vi "SISE-Monitor110.vi"() -> ()   [LabVIEW 2024]
uses:
  Labview-Projects2019/IonFluxProgramms2019/IonFluxMonitor/SubVIs-SISE-Monitor/Control-IonFlux.ctl
  <vilib>/DAQmx/read.llb/DAQmx Read (Analog 2D DBL NChan NSamp).vi
  <vilib>/Instr/_visa.llb/VISA Configure Serial Port (Instr).vi
  <vilib>/DAQmx/create/channels.llb/DAQmx Create Channel (AI-Voltage-Basic).vi
  <vilib>/DAQmx/miscellaneous.llb/DAQmx Fill In Error Info.vi
  <vilib>/Analysis/NI_AALPro.lvlib
panel:
  out "Lesepuffer":string
  out "Registerkarte":enum32{"Start", "Record", "Stop"}(tab)
  out "Output V ch 2":bool
  in  "V channel 2":bool
  out "Output V ch 1":bool
  in  "V channel 1":bool
  out "SISE channel 1":bool
  out "Output SISE ch 2":bool
  in  "SISE channel 2":bool
  out "slow":bool
  in  "Scan angle (degrees)":dbl(slide) scale=0.0..90.0
  out "?":dbl
  in  "VISA res. name":refnum<visa-resource-name> caption="VISA-Ressourcenname"
  in  "Start measurement":bool
  out "Data File":bool
  out "Ind. Channel In":bool
  in  "Data file":path
  out "Ind. Channel Out":bool
  out "?":dbl
  out "Record period (round at 5s)":dbl
  in  "Scan distance (µm)":dbl(slide)=50.0 scale=0.0..100.0
  in  "Record period (single track, s)":dbl(slide)=10.112359550561797 scale=0.0..60.0 scale format="%#_2f"
  in  "Manipulator Speed":bool
  out "fast":bool
  in  "Channels In":tag
  in  "Position of manipulator":bool=TRUE
  out "right":bool
  out "left":bool
  in  "TC 3":T1(tab)
  in  "Range limit\nS1.1 (mV)":dbl(slide)=200.0 min=0.0 max=600.0 scale=0.2..600.0
  in  "Base line\nS1.1 (mV)":dbl(slide) scale=-300.0..300.0
  in  "Range limit\nS1.2 mV":dbl(slide)=30.0 scale=0.1..30.0
  in  "Base line \nS1.2 (mV)":dbl(slide) scale=-15.0..15.0
  out "dV-SISE channel 1":cluster{dbl[], dbl[]}[](graph)
  out "V-SISE channel 1":cluster{dbl[], dbl[]}[](graph)
  out "V-SISE channel 2":cluster{dbl[], dbl[]}[](graph)
  out "dV-SISE channel 2":cluster{dbl[], dbl[]}[](graph)
  in  "Range limit\nS2.1 (mV)":dbl(slide)=200.0 min=0.0 max=600.0 scale=0.2..600.0
  in  "Base line\nS2.1 (mV)":dbl(slide) scale=-300.0..300.0
  in  "Base line \nS2.2 (mV)":dbl(slide) scale=-15.0..15.0
  in  "Range limit\nS2.2 (mV)":dbl(slide)=30.0 scale=0.1..30.0
  out "Voltage channel 1":cluster{dbl[], dbl[]}[](graph)
  in  "Base line\nV1 (V)":dbl(slide) scale=-10.0..10.0
  in  "Range limit\nV1 (V)":dbl(slide)=24.63054187192118 min=0.0 max=600.0 scale=0.0..25.0
  in  "Base line\nV2 (V)":dbl(slide) scale=-10.0..10.0
  in  "Range limit\nV2 (V)":dbl(slide)=24.63054187192118 min=0.0 max=600.0 scale=0.0..25.0
  out "Voltage channel 2":cluster{dbl[], dbl[]}[](graph)
  out "V channel #2":bool
  out "V channel #1":bool
  out "SISE channel #2":bool
  out "SISE channel #1":bool
  in  "?":T2(tab)
  out "Vprobe SISE 1":cluster{dbl[], dbl[]}[](graph)
  out "Vprobe SISE 2":cluster{dbl[], dbl[]}[](graph)
  out "Vprobe V 1":cluster{dbl[], dbl[]}[](graph)
  out "Vprobe V 2":cluster{dbl[], dbl[]}[](graph)
  in  "Enable change position 0":bool
  out "Raw data file":path
  in  "Stop measurent":bool
  out "Position probe":cluster{dbl[], dbl[]}[](graph)
  in  "Add Mark":bool
  in  "Event Mark":string
  out "Stop recording":bool
  out "String":string
  out "E-mark on":T3
  out "?":string
  in  "Bildlaufleiste":i32(c297)
  in  "Start fit (% of rec. period)":dbl(slide)=50.0 scale=0.0..100.0
  in  "?":enum32{"dV SISE 1", "dV SISE 2"}(tab)
  out "deltaV SISE 1":cluster{dbl[], "Best Linear Fit":dbl[]}[](graph)
  out "deltaV SISE 2":cluster{dbl[], "Best Linear Fit":dbl[]}[](graph)
  in  "Zoom from start":dbl(slide) scale=0.0..100.0
  in  "Zoom from end":dbl(slide)=100.0 scale=0.0..100.0
  in  "Stop programm":bool
  in  "New measurement":bool
  out "Stop recording 2":bool
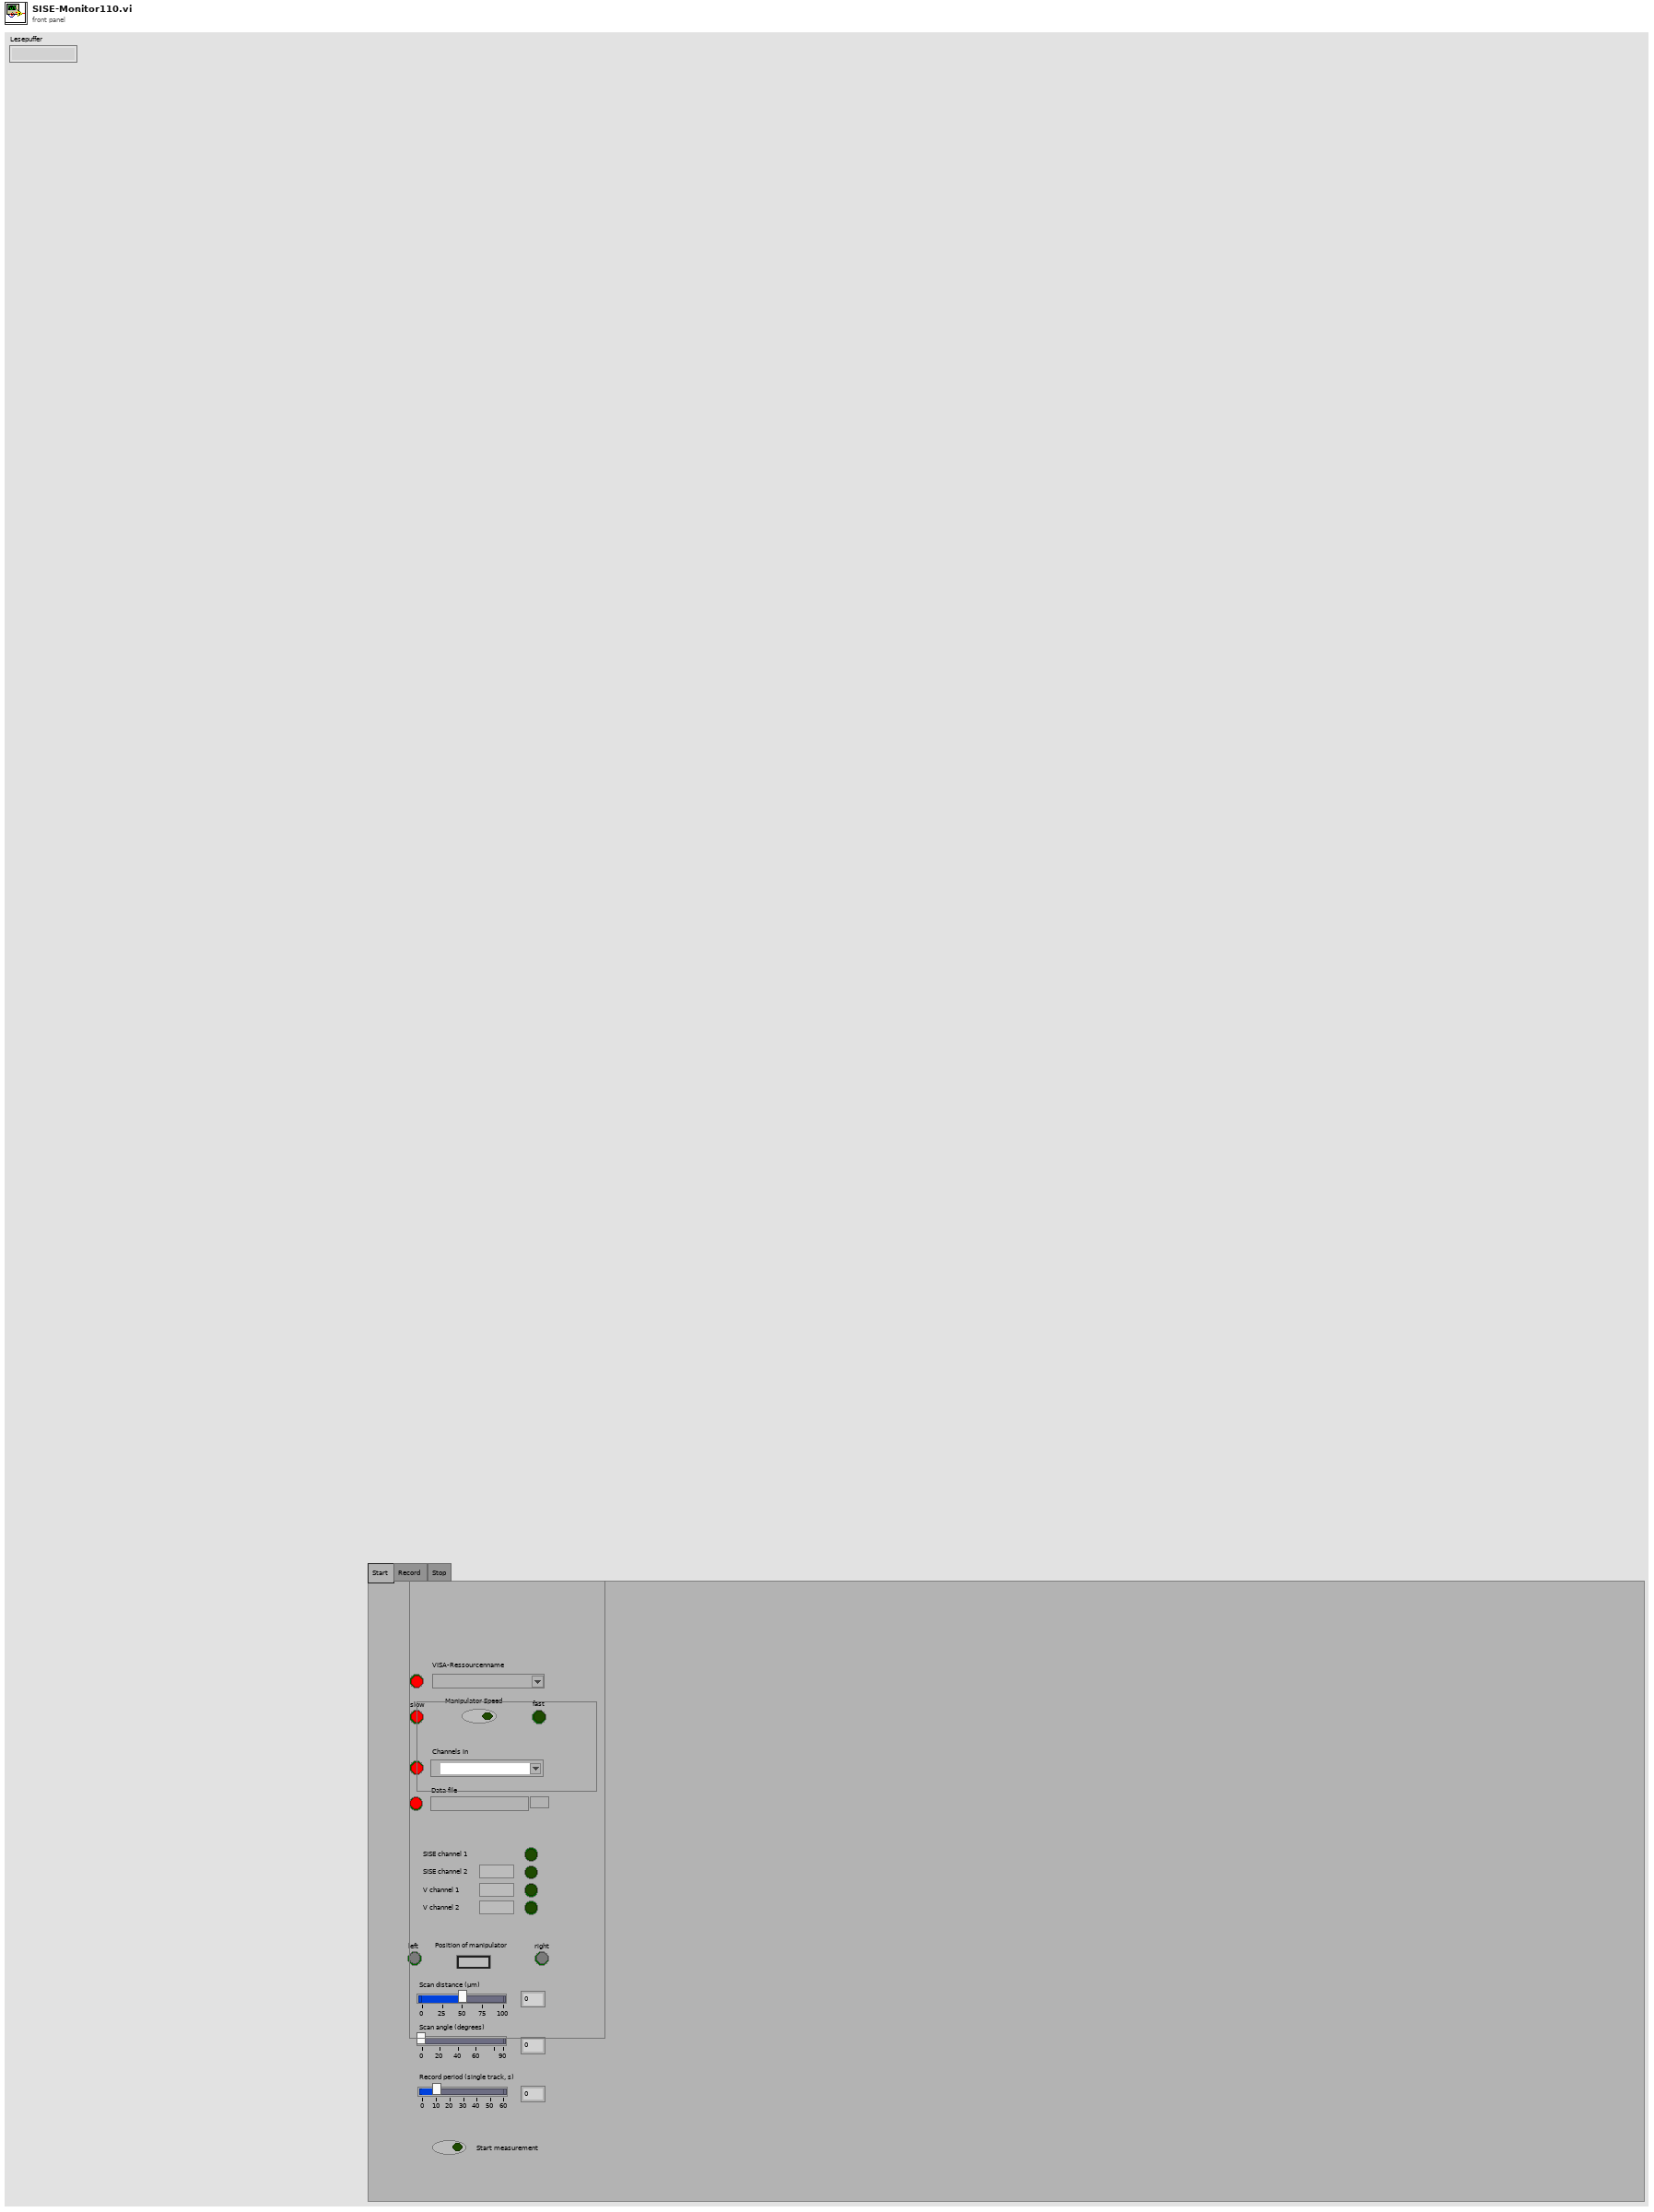
[diagram p1: front panel]
types:
  T1 = enum32{"SISE channel #1", "SISE channel #2", "V channel #1", "V channel #2"}
  T2 = enum32{"SISE chan #1", "SISE chan #2", "V chan #1", "V chan #2"}
  T3 = typedef "Control-IonFlux.ctl" = bool
  T4 = cluster{"refnum out":refnum<file>, "status":bool, "code":i32, "source":string}
  T5 = cluster{"task out":refnum<k21>, "status":bool, "code":i32, "source":string}
  T6 = enum16{"open", "replace", "create", "open or create", "replace or create", "replace or create with confirmation"}
  T7 = cluster{"refnum":refnum<file>, "status":bool, "code":i32, "source":string}
  T8 = cluster{dbl[], dbl[], "Best Linear Fit":dbl[], dbl[], dbl[]}
  T9 = cluster{"Array (Ausgang)":dbl[], "Array (Ausgang)":dbl[]}
  T10 = cluster{"Array (Ausgang)":dbl[], "Array (Ausgang)":dbl[]}[]
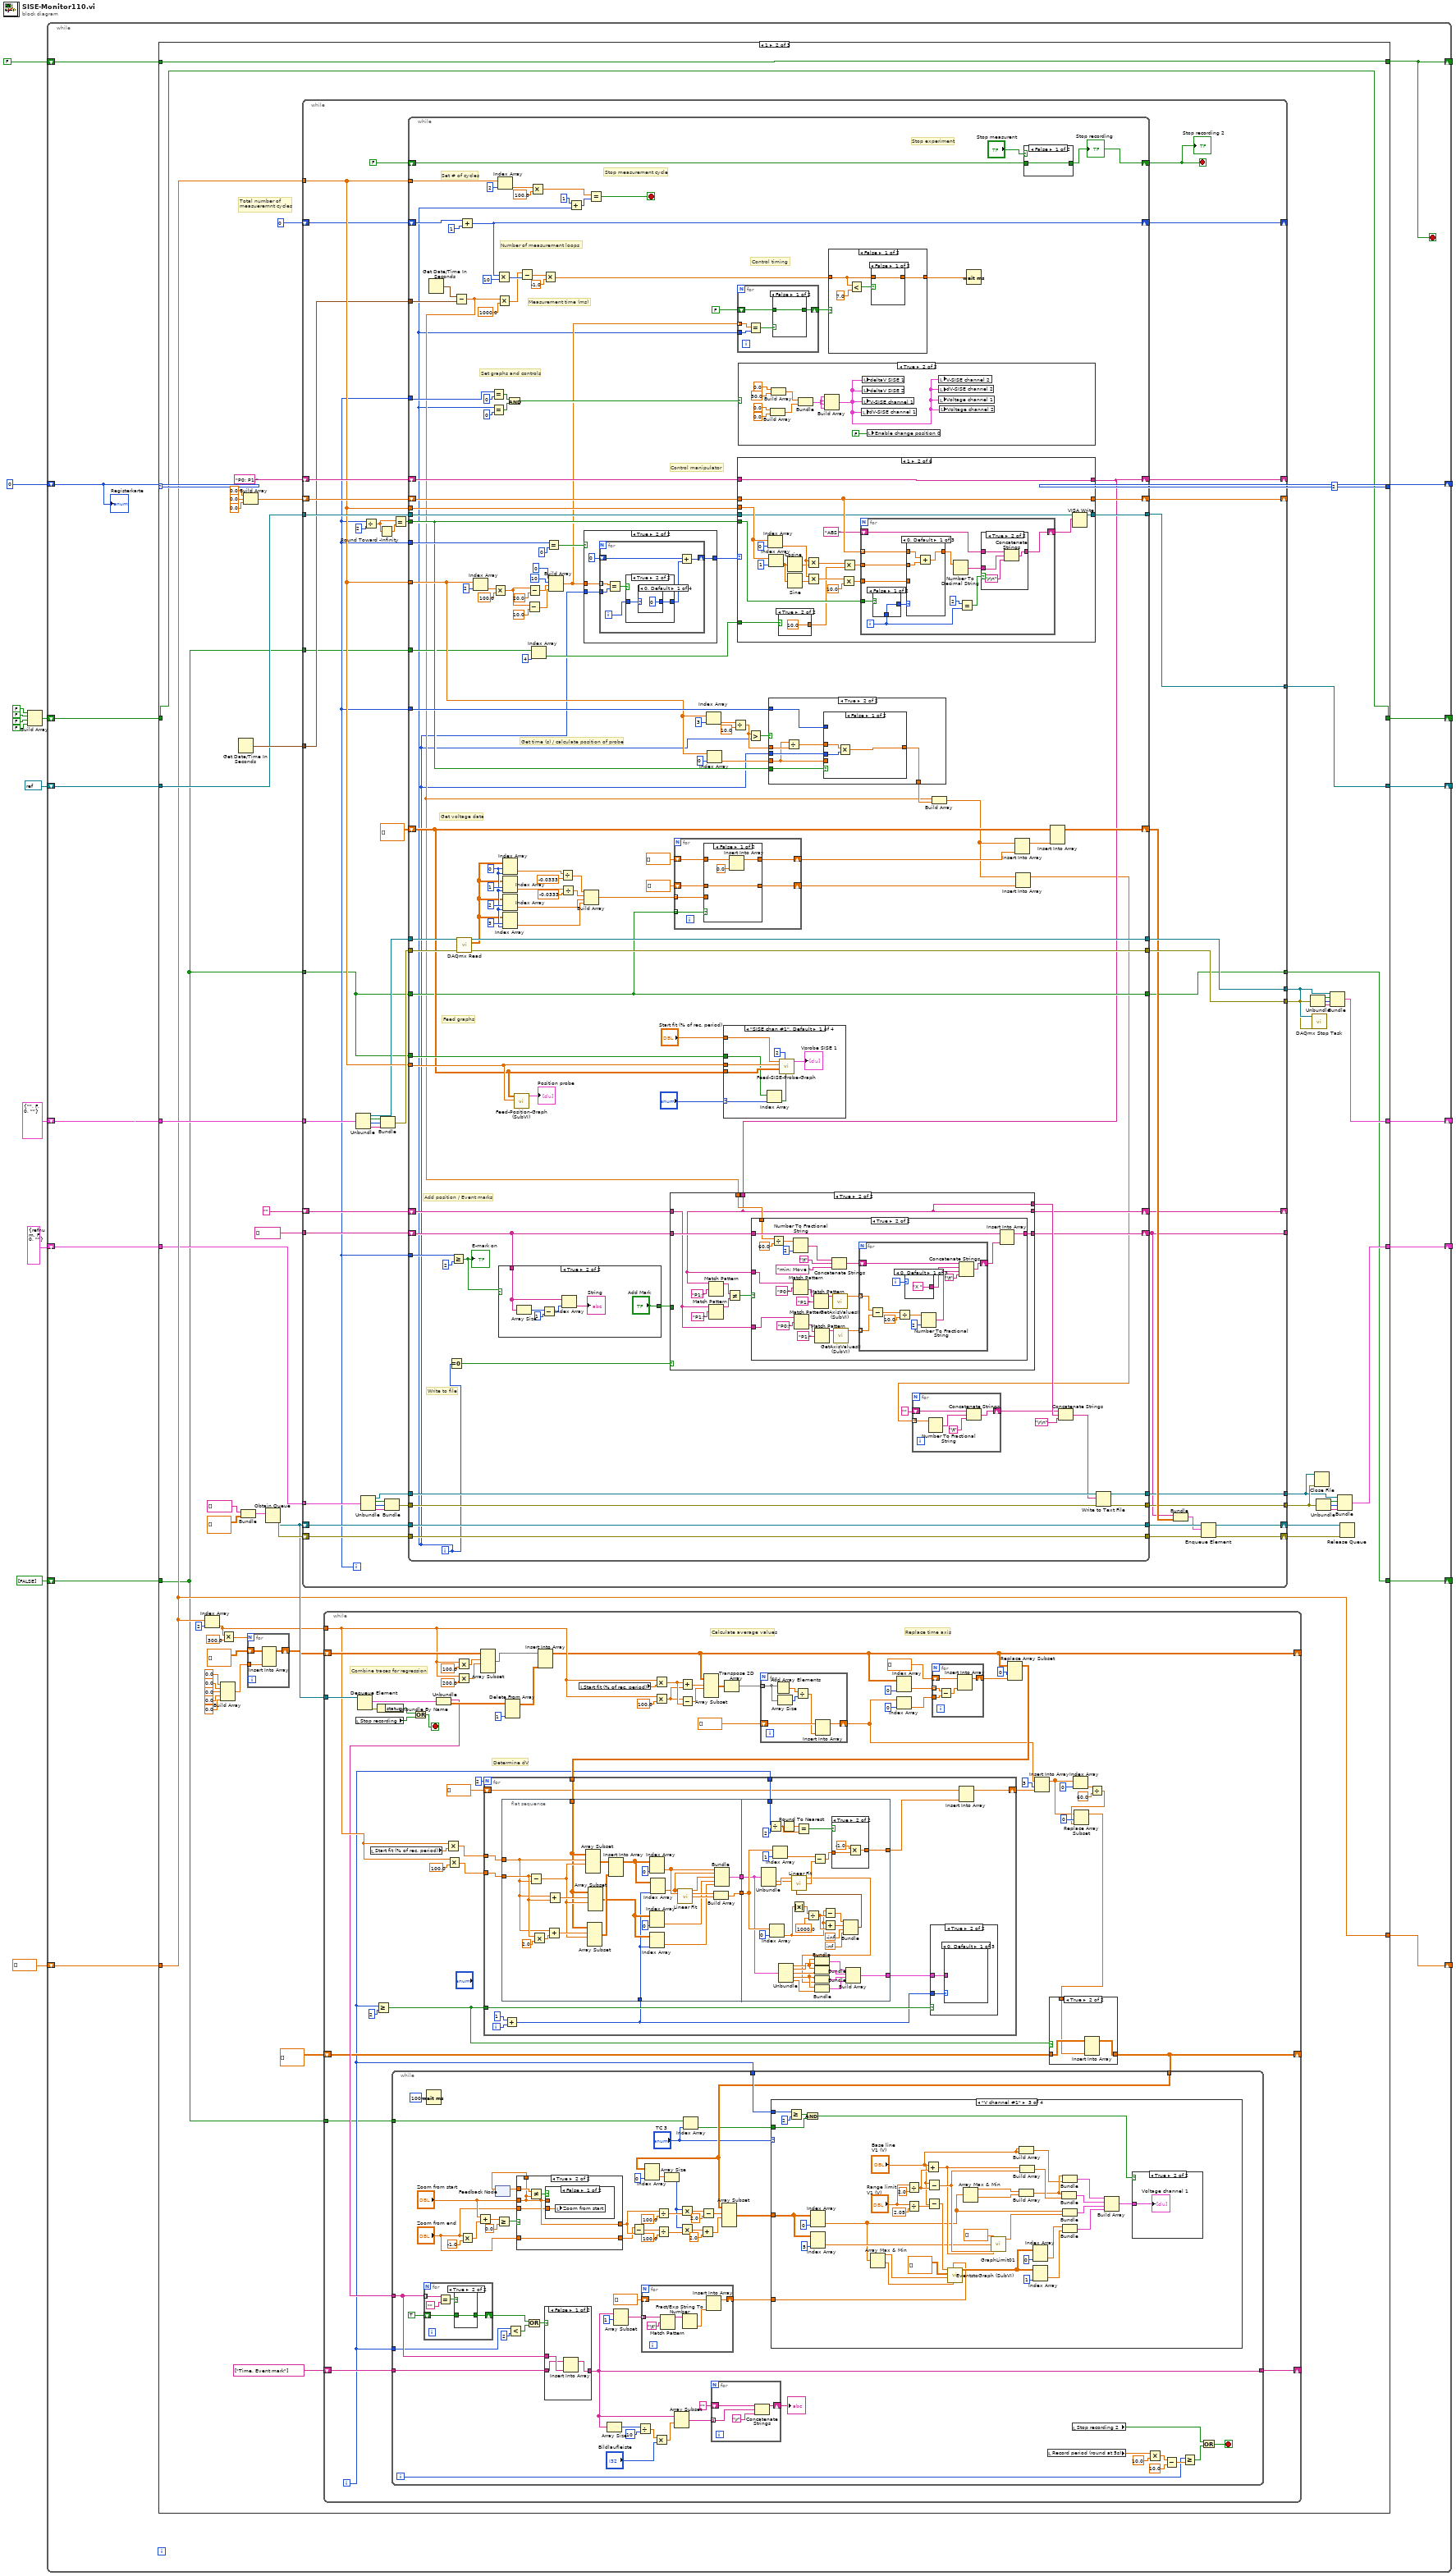
[diagram p0: block diagram]
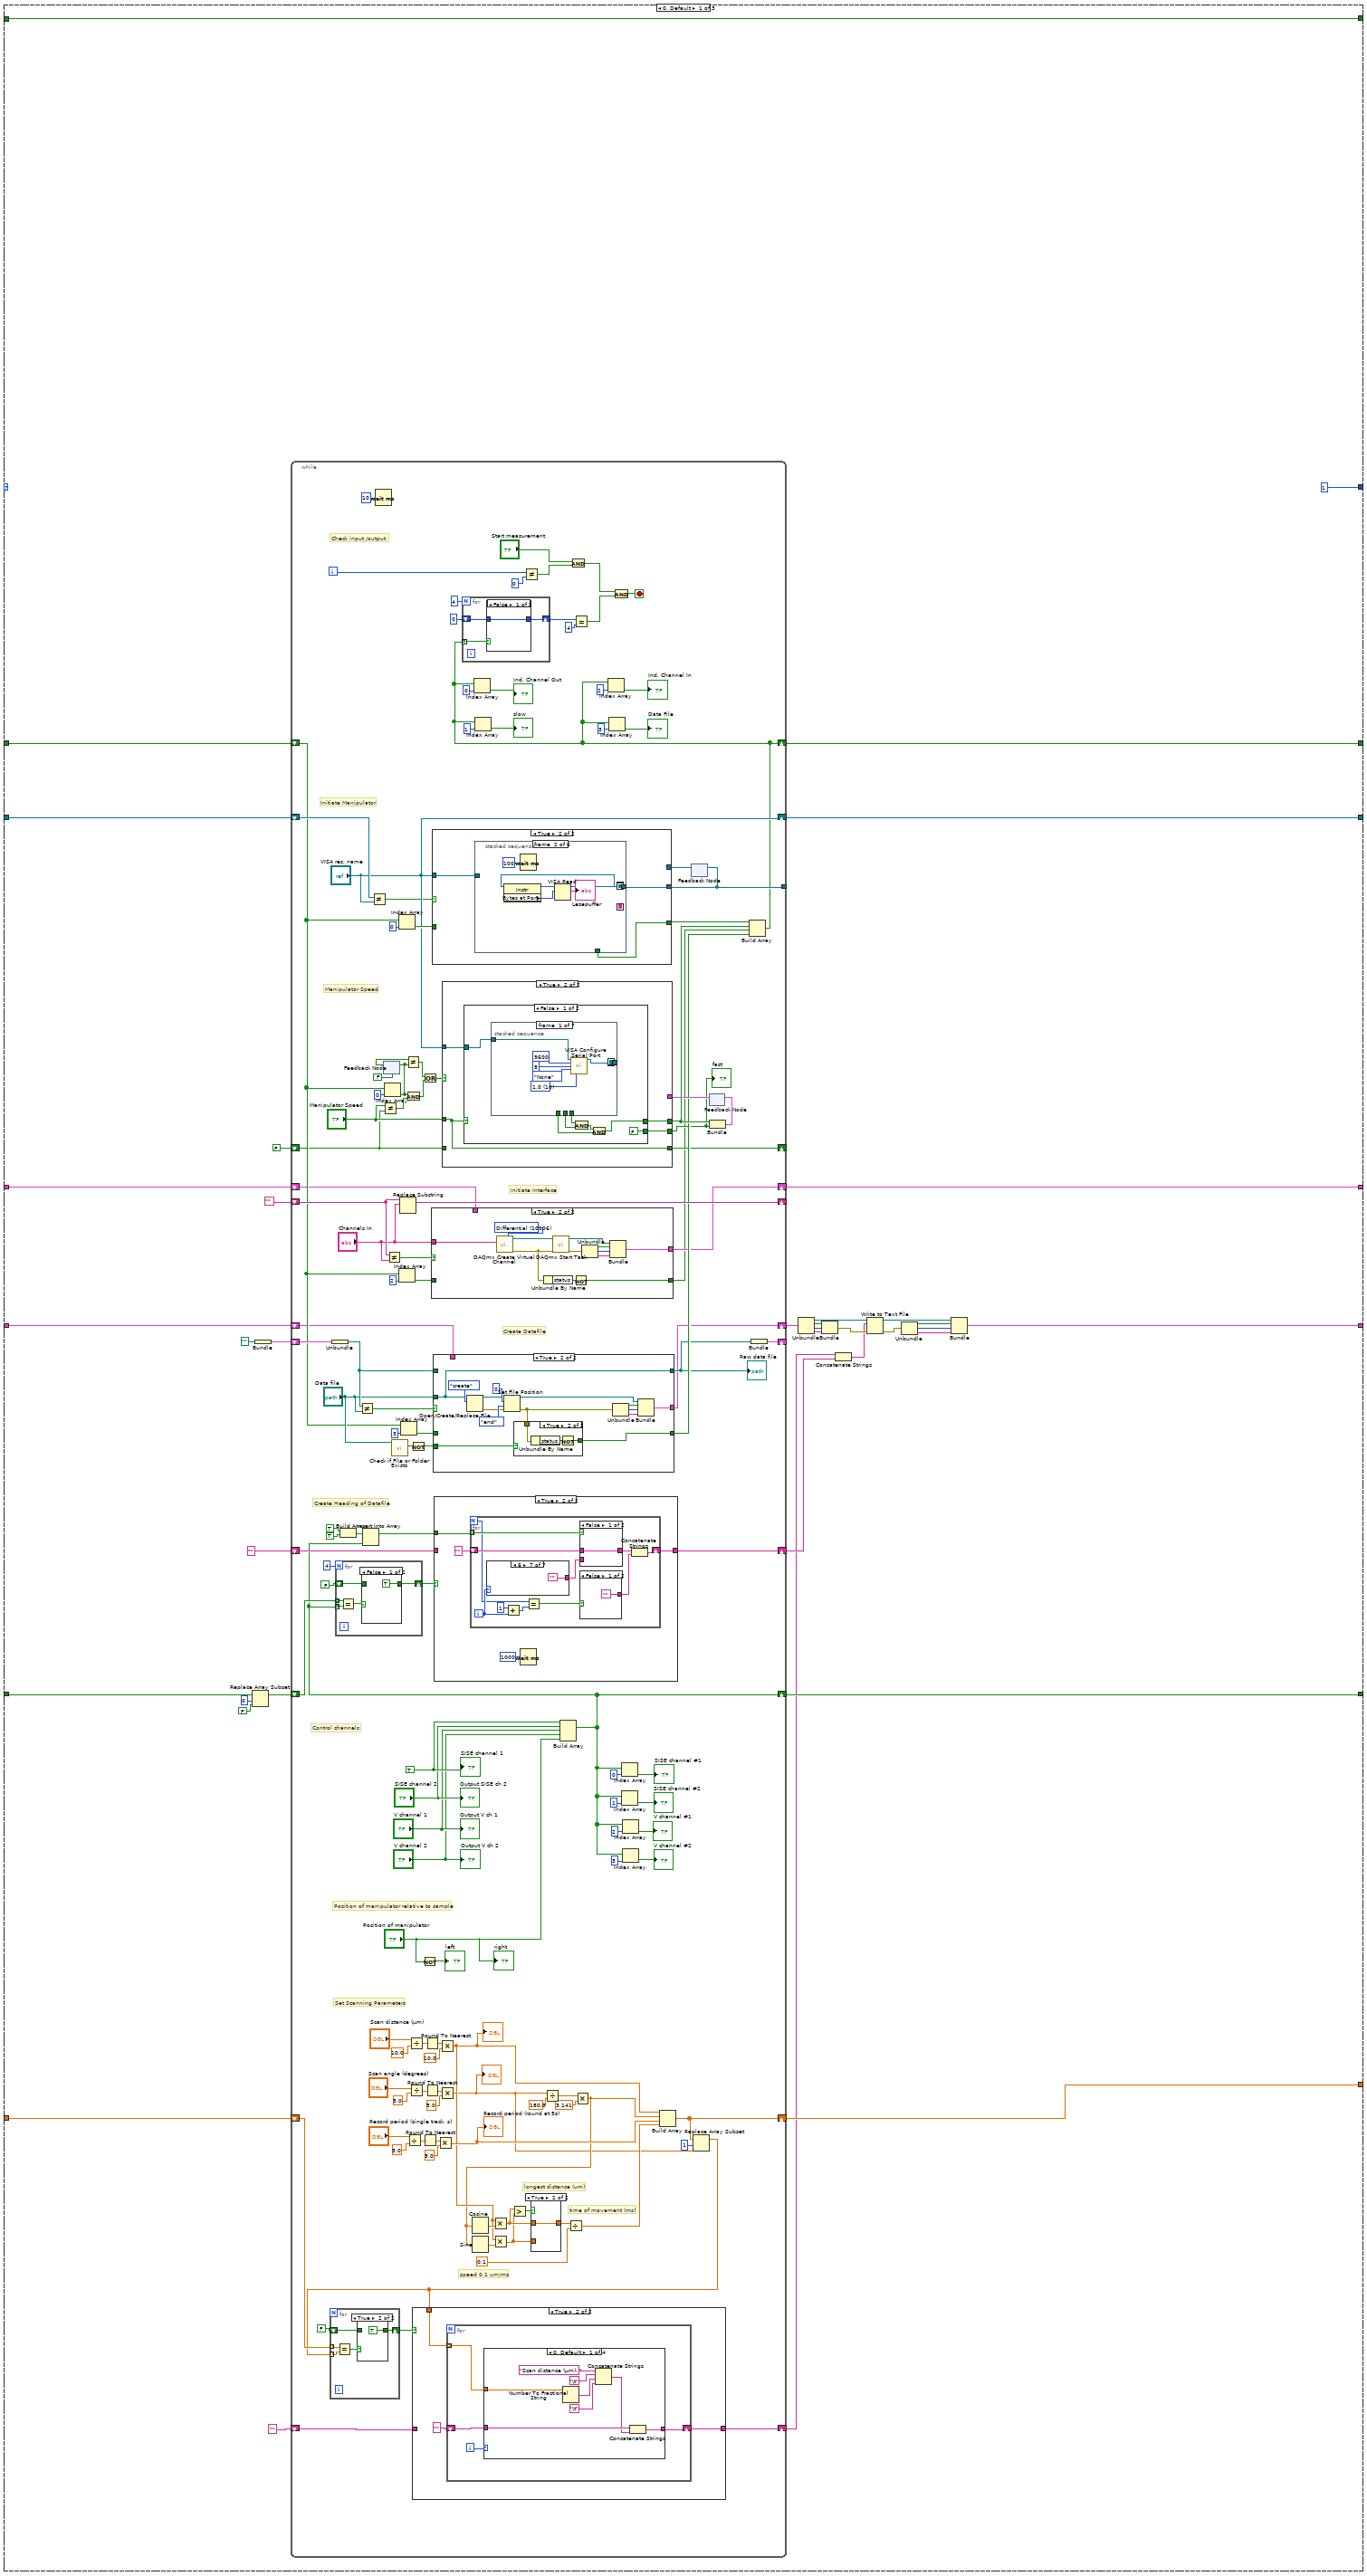
[diagram p2: hidden frame]
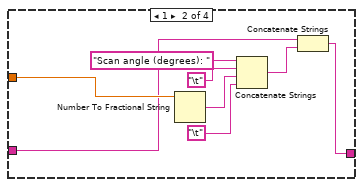
[diagram p4: hidden frame]
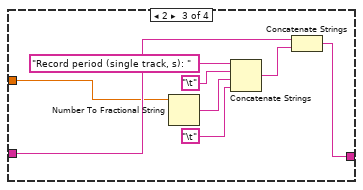
[diagram p5: hidden frame]
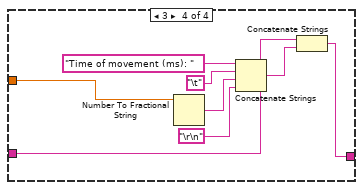
[diagram p6: hidden frame]
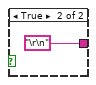
[diagram p10: hidden frame]
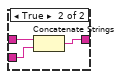
[diagram p11: hidden frame]
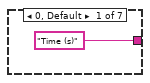
[diagram p12: hidden frame]
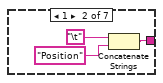
[diagram p13: hidden frame]
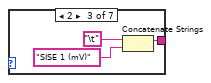
[diagram p14: hidden frame]
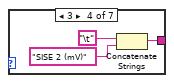
[diagram p15: hidden frame]
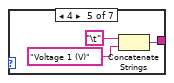
[diagram p16: hidden frame]
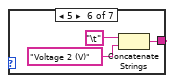
[diagram p17: hidden frame]
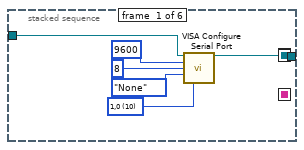
[diagram p19: hidden frame]
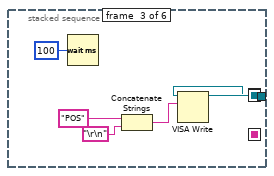
[diagram p20: hidden frame]
diagram:
  n1 = Build Array(FALSE, FALSE, FALSE, FALSE) -> (w1:bool[])
  n2 = while {
    shift-right: [w28] -> _
    shift-left: 0 -> [w27]
    shift-right: [w25] -> _
    shift-left: refnum<visa-resource-name> refnum ("VISA res. name") -> [w26]
    shift-right: [w23] -> _
    shift-left: T5 {"task out"="", "status"=FALSE, "code"=0, "source"=""} -> [w24]
    shift-right: [w19] -> _
    shift-left: T4 {"refnum out"=refnum, "status"=FALSE, "code"=0, "source"=""} -> [w20]
    shift-right: [w22] -> _
    shift-left: dbl[] [] -> [w21]
    shift-right: [w18] -> _
    shift-left: bool[] [FALSE] -> [w17]
    shift-right: [w15] -> _
    shift-left: FALSE -> [w16]
    shift-right: [w13] -> _
    shift-left: w1 -> [w14]
    stop <- w15 stop-if-true
    n3 = case shown="1" w27 {
      tunnel: [1 2 0] -> w28
      tunnel: w26 -> [w60 w557 w1623]
      tunnel: [w59 w556 w1623] -> w25
      tunnel: w24 -> [w58 w555 w1622]
      tunnel: [w57 w551 w1622] -> w23
      tunnel: [w40 w530 w1620] -> w19
      tunnel: w20 -> [w56 w534 w1620]
      tunnel: [w55 w544 w1621] -> w22
      tunnel: w21 -> [w54 w544 w1621]
      tunnel: w17 -> [w31 w513 w1619]
      tunnel: [w53 w527 w1619] -> w18
      tunnel: w16 -> [w39 w520 w1618]
      tunnel: [w39 w520 w1617] -> w15
      tunnel: w14 -> [w33 w519 w1616]
      tunnel: [w38 w519 w1616] -> w13
      frame 0, Default {
        n4 = Replace Array Subset(array=w31, new element=FALSE ("Neues Element/Teil-Array"), index=0 ("Index")) -> (w32:bool[])
        n5 = Bundle(path "") -> (w61:cluster{path})  [unwired: 1 in]
        n6 = while {
          shift-right: ["VISA res. name"] -> w59
          shift-left: w60 -> [w184]
          shift-right: [w91] -> w38
          shift-left: w33 -> [w138]
          tunnel: [w140] -> _
          shift-right: [w179] -> _
          shift-left: "" -> [w178]
          shift-right: [w169] -> _
          shift-left: w61 -> [w171]
          shift-right: [w120] -> _
          shift-left: FALSE -> [w135]
          shift-right: [w117] -> w57
          shift-left: w58 -> [w118]
          shift-right: [w115] -> w51
          shift-left: w56 -> [w114]
          shift-right: [w74] -> w55
          shift-left: w54 -> [w78]
          shift-right: [w67] -> w53
          shift-left: w32 -> [w86]
          shift-right: [w88] -> w36
          shift-left: "" -> [w87]
          shift-right: [w80] -> w35
          shift-left: "" -> [w76]
          i -> [w82]
          stop <- w84 stop-if-true
          w110 = TRUE
          # "Position of manipulator relative to sample"
          # "Set Scanning Parameters"
          # "Control channels"
          # "Create Heading of Datafile"
          # "Create Datafile"
          # "Initiate Interface"
          # "Manipulator Speed"
          # "Initiate Manipulator"
          # "Check input /output"
          # "speed 0.1 um/ms"
          # "longest distance (um)"
          # "time of movement (ms)"
          n7 = Unbundle(w171) -> (w170:path)
          n8 = Build Array(TRUE, TRUE) -> (w95:bool[])
          n9 = Not Equal?(x=w170, y="Data file") -> (x != y?=w94:bool)
          n10 = Not Equal?(x=w184, y="VISA res. name") -> (x != y?=w81:bool)
          n11 = Wait (ms)(milliseconds to wait=u32 10) -> ()  [unwired: 1 out]
          n12 = Not Equal?(x="Manipulator Speed", y=w135) -> (x != y?=w137:bool)
          n13 = feedback #1(FALSE) -> (w132:bool)
          n14 = Index Array(array=w138, index=0 ("Index")) -> (element=w133:bool)
          n15 = feedback-in #1(w133) -> ()
          n16 = Not Equal?(x=w178, y="Channels In") -> (x != y?=w181:bool)
          n17 = call <vilib>:"Check if File or Folder Exists.vi"("path"="Data file") -> ("file or folder exists?"=w175:bool)  [unwired: 8 in, 2 out]
          n18 = Index Array(array=w138, index=2 ("Index")) -> (element=w180:bool)
          n19 = Index Array(array=w138, index=0 ("Index")) -> (element=w144:bool)
          n20 = Replace Substring(4:"Channels In", 5:w178) -> (1:w179:string)  [unwired: 2 in, 1 out]
          n21 = Index Array(array=w138, index=3 ("Index")) -> (element=w172:bool)
          n22 = Not Equal?(x=w132, y=w133) -> (x != y?=w131:bool)
          n23 = And(x=w133, y=w137) -> (x .and. y?=w129:bool)
          n24 = Divide(x="Record period (single track, s)", y=5.0) -> (x/y=w185:dbl)
          n25 = Divide(x="Scan distance (µm)", y=10.0) -> (x/y=w192:dbl)
          n26 = Divide(x="Scan angle (degrees)", y=5.0) -> (x/y=w159:dbl)
          n27 = Not(x=w175) -> (.not. x?=w167:bool)
          n28 = Not(x="Position of manipulator") -> (.not. x?=→"left":bool)
          n29 = Round To Nearest(number=w185) -> (nearest integer value=w188:dbl)
          n30 = Or(x=w131, y=w129) -> (x .or. y?=w130:bool)
          n31 = Round To Nearest(number=w192) -> (nearest integer value=w191:dbl)
          n32 = Round To Nearest(number=w159) -> (nearest integer value=w158:dbl)
          n33 = case shown="True" w181 {
            tunnel: w180 -> [w370 _]
            tunnel: [w370 w381] -> w70
            tunnel: "Channels In" -> [_ w372]
            tunnel: w118 -> [w369 _]
            tunnel: [w369 w375] -> w117
            frame False {
            }
            frame True {
              w371 = 10106 items=["Default"=-1, "RSE"=10083, "NRSE"=10078, "Differential"=10106, "Pseudodifferential"=12529] ("input terminal configuration")
              n34 = call-poly <vilib>:"DAQmx Create Virtual Channel.vi"("input terminal configuration"=w371, "physical channels"=w372) -> ("task out"=w374:refnum<k21>, "error out"=w373:errorcluster)  [unwired: 12 in]
              n35 = Unbundle By Name(w373) -> ("status"=w382:bool)
              n36 = call <vilib>:"DAQmx Start Task.vi"("task/channels in"=w374, "error in"=w373) -> ("task out"=w376:refnum<k21>, "error out"=w380:errorcluster)  [unwired: 12 in]
              n37 = Not(x=w382) -> (.not. x?=w381:bool)
              n38 = Unbundle(w380) -> ("status"=w377:bool, "code"=w378:i32, "source"=w379:string)
              n39 = Bundle("task out"=w376, "status"=w377, "code"=w378, "source"=w379) -> (w375:T5)  [unwired: 1 in]
            }
          }
          n40 = case shown="True" w94 {
            tunnel: "Data file" -> [_ w358]
            tunnel: [w350 w359] -> w121
            tunnel: w172 -> [w350 _]
            tunnel: w170 -> [w349 _]
            tunnel: [w349 w358] -> w116
            tunnel: w167 -> [_ w357]
            tunnel: [w348 w353] -> w115
            tunnel: w114 -> [w348 _]
            frame False {
            }
            frame True {
              n41 = Open/Create/Replace File(file path (use dialog)=w358, operation (0:open)=T6."create") -> (refnum out=w362:refnum<file>, error out=w361:errorcluster)  [unwired: 4 in, 1 out]
              n42 = Set File Position(offset (in bytes) (0)=i64 0, refnum=w362, from (0:start)=enum16{"start", "end", "current"}."end", error in=w361) -> (refnum out=w351:refnum<file>, error out=w352:errorcluster)
              n43 = case shown="True" w357 {
                tunnel: [FALSE w367] -> w359
                tunnel: w352 -> [_ w366]
                frame False {
                }
                frame True {
                  n44 = Unbundle By Name(w366) -> ("status"=w368:bool)
                  n45 = Not(x=w368) -> (.not. x?=w367:bool)
                }
              }
              n46 = Unbundle(w352) -> ("status"=w356:bool, "code"=w355:i32, "source"=w354:string)
              n47 = Bundle("refnum"=w351, "status"=w356, "code"=w355, "source"=w354) -> (w353:T7)  [unwired: 1 in]
            }
          }
          "Raw data file" <- w116
          n48 = Multiply(x=w188, y=5.0) -> (x*y=w154:dbl)
          "Record period (round at 5s)" <- w154
          n49 = Multiply(x=w191, y=10.0) -> (x*y=w148:dbl)
          "?" <- w148
          n50 = Multiply(x=w158, y=5.0) -> (x*y=w72:dbl)
          "?" <- w72
          n51 = Not Equal?(x=w82, y=0) -> (x != y?=w164:bool)
          n52 = Divide(x=w72, y=180.0) -> (x/y=w111:dbl)
          n53 = Build Array(w110, "SISE channel 2", "V channel 1", "V channel 2", "Position of manipulator") -> (w67:bool[])
          n54 = for {
            N: 4 -> [_]
            tunnel: w86 -> [w247] mode=indexing
            tunnel: w67 -> [w246] mode=indexing
            shift-right: [w243] -> w83
            shift-left: FALSE -> [w244]
            n55 = Equal?(x=w247, y=w246) -> (x = y?=w245:bool)
            n56 = case shown="False" w245 {
              tunnel: w244 -> [_ w249]
              tunnel: [TRUE w249] -> w243
              frame False {
              }
              frame True {
              }
            }
          }
          n57 = Insert Into Array(array=w95, new element=w67) -> (w89:bool[])  [unwired: 1 in]
          n58 = case shown="True" w83 {
            tunnel: w89 -> [_ w253]
            tunnel: [w250 w252] -> w88
            tunnel: w87 -> [w250 _]
            frame False {
            }
            frame True {
              n59 = for {
                N -> [w257]
                shift-right: [w262] -> w252
                shift-left: "" -> [w265]
                tunnel: w253 -> [w263] mode=indexing
                i -> [w260]
                n60 = case shown="6" w260 {
                  tunnel: ["Time (s)" w275 w278 w281 w284 w287 ""] -> w264
                  frame 0, Default {
                  }
                  frame 1 {
                    n61 = Concatenate Strings("\t", "Position") -> (w275:string)
                  }
                  frame 2 {
                    n62 = Concatenate Strings("\t", "SISE 1 (mV)") -> (w278:string)
                  }
                  frame 3 {
                    n63 = Concatenate Strings("\t", "SISE 2 (mV)") -> (w281:string)
                  }
                  frame 4 {
                    n64 = Concatenate Strings("\t", "Voltage 1 (V)") -> (w284:string)
                  }
                  frame 5 {
                    n65 = Concatenate Strings("\t", "Voltage 2 (V)") -> (w287:string)
                  }
                  frame 6 {
                  }
                }
                n66 = Add(x=1, y=w260) -> (x+y=w258:i32)
                n67 = Equal?(x=w257, y=w258) -> (x = y?=w256:bool)
                n68 = case shown="False" w263 {
                  tunnel: w265 -> [w268 w271]
                  tunnel: [w268 w270] -> w261
                  tunnel: w264 -> [_ w269]
                  frame False {
                  }
                  frame True {
                    n69 = Concatenate Strings(w271, w269) -> (w270:string)
                  }
                }
                n70 = case shown="False" w256 {
                  tunnel: ["" "\r\n"] -> w255
                  frame False {
                  }
                  frame True {
                  }
                }
                n71 = Concatenate Strings(w261, w255) -> (w262:string)
              }
              n72 = Wait (ms)(milliseconds to wait=u32 1000) -> ()  [unwired: 1 out]
            }
          }
          n73 = And(x="Start measurement", y=w164) -> (x .and. y?=w90:bool)
          n74 = Multiply(x=w111, y=3.141) -> (x*y=w75:dbl)
          n75 = Cosine(x=w75) -> (cos(x)=w153:dbl)
          n76 = Sine(x=w75) -> (sin(x)=w152:dbl)
          n77 = Multiply(x=w148, y=w153) -> (x*y=w151:dbl)
          n78 = Multiply(x=w148, y=w152) -> (x*y=w150:dbl)
          n79 = Greater?(x=w151, y=w150) -> (0:w149:bool)
          n80 = case shown="True" w149 {
            tunnel: w151 -> [_ w340]
            tunnel: w150 -> [w339 _]
            tunnel: [w339 w340] -> w147
            frame False {
            }
            frame True {
            }
          }
          n81 = Divide(x=w147, y=0.1) -> (x/y=w145:dbl)
          n82 = Index Array(array=w67, index=0 ("Index")) -> (element=→"SISE channel #1":bool)
          n83 = Index Array(array=w67, index=1 ("Index")) -> (element=→"SISE channel #2":bool)
          n84 = Index Array(array=w67, index=2 ("Index")) -> (element=→"V channel #1":bool)
          n85 = Index Array(array=w67, index=3 ("Index")) -> (element=→"V channel #2":bool)
          n86 = Build Array(w148, w75, w154, w145) -> (w74:dbl[])
          n87 = feedback #2() -> (w143:refnum<visa-resource-name>)  [unwired: 1 in]
          n88 = case shown="True" w81 {
            tunnel: w144 -> [w290 _]
            tunnel: [w290 w293] -> w128
            tunnel: "VISA res. name" -> [_ w292]
            tunnel: [w289 w291] -> w140
            tunnel: w143 -> [w289 _]
            frame False {
            }
            frame True {
              n89 = stacked-sequence {
                seq-local: [w294 _ _ _ _ _] -> [_ w301 _ _ _ _]
                seq-local: [_ w302 _ _ _ _] -> [_ _ w306 _ _ _]
                seq-local: [_ _ w307 _ _ _] -> [_ _ _ w314 _ _]
                seq-local: [_ _ _ w313 _ _] -> [_ _ _ _ w325 _]
                seq-local: [_ _ _ w312 _ _] -> [_ _ _ _ w319 _]
                seq-local: [_ _ _ _ w324 _] -> [_ _ _ _ _ w335]
                tunnel: w292 -> [w299 _ _ _ _ _]
                tunnel: [_ _ _ _ _ w334] -> w291
                tunnel: [_ _ _ _ _ w329] -> w293
                frame #0 {
                  w295 = u16 10 items=["1,0"=10, "1,5"=15, "2,0"=20] ("stop bits (10: 1 bit)")
                  n90 = call-poly "VISA Configure Serial Port"("VISA resource name"=w299, "baud rate (9600)"=u32 9600, "data bits (8)"=u16 8, "parity (0:none)"=enum16{"None", "Odd", "Even", "Mark", "Space"}."None", "stop bits (10: 1 bit)"=w295) -> ("VISA resource name out"=w294:refnum<visa-resource-name>)  [unwired: 9 in, 1 out]
                }
                frame #1 {
                  n91 = property class="Instr"(reference=w301) -> (reference out=w304:refnum<visa-resource-name>, "Bytes at Port"=w303:u32)  [unwired: 1 in, 1 out]
                  n92 = Wait (ms)(milliseconds to wait=u32 100) -> ()  [unwired: 1 out]
                  n93 = VISA Read(VISA resource name=w304, byte count=w303) -> (VISA resource name out=w302:refnum<visa-resource-name>, read buffer=→"Lesepuffer":string)  [unwired: 1 in, 2 out]
                }
                frame #2 {
                  n94 = Wait (ms)(milliseconds to wait=u32 100) -> ()  [unwired: 1 out]
                  n95 = Concatenate Strings("POS", "\r\n") -> (w308:string)
                  n96 = VISA Write(VISA resource name=w306, write buffer=w308) -> (VISA resource name out=w307:refnum<visa-resource-name>)  [unwired: 1 in, 2 out]
                }
                frame #3 {
                  n97 = property class="Instr"(reference=w314) -> (reference out=w315:refnum<visa-resource-name>, "Bytes at Port"=w316:u32)  [unwired: 1 in, 1 out]
                  n98 = Wait (ms)(milliseconds to wait=u32 100) -> ()  [unwired: 1 out]
                  n99 = VISA Read(VISA resource name=w315, byte count=w316) -> (VISA resource name out=w313:refnum<visa-resource-name>, read buffer=w312:string)  [unwired: 1 in, 2 out]
                }
                frame #4 {
                  n100 = String Length(string=w319) -> (length=w322:i32)
                  n101 = Subtract(x=w322, y=1) -> (x-y=w320:i32)
                  n102 = Wait (ms)(milliseconds to wait=u32 100) -> ()  [unwired: 1 out]
                  n103 = String Subset(string=w319, length (rest)=w320) -> (substring=w318:string)  [unwired: 1 in]
                  n104 = Concatenate Strings("ABS ", w318, "\r\n") -> (w326:string)
                  n105 = VISA Write(VISA resource name=w325, write buffer=w326) -> (VISA resource name out=w324:refnum<visa-resource-name>)  [unwired: 1 in, 2 out]
                }
                frame #5 {
                  n106 = property class="Instr"(reference=w335) -> (reference out=w336:refnum<visa-resource-name>, "Bytes at Port"=w337:u32)  [unwired: 1 in, 1 out]
                  n107 = Wait (ms)(milliseconds to wait=u32 100) -> ()  [unwired: 1 out]
                  n108 = VISA Read(VISA resource name=w336, byte count=w337) -> (VISA resource name out=w334:refnum<visa-resource-name>, read buffer=w330:string)  [unwired: 1 in, 2 out]
                  n109 = Concatenate Strings("A", "\r") -> (w333:string)
                  n110 = Equal?(x=w330, y=w333) -> (x = y?=w329:bool)
                }
              }
            }
          }
          n111 = feedback-in #2(w140) -> ()
          n112 = Replace Array Subset(array=w74, new element=w72, index=1 ("Index")) -> (w71:dbl[])
          n113 = for {
            shift-right: [w236] -> w77
            shift-left: FALSE -> [w237]
            tunnel: w78 -> [w240] mode=indexing
            tunnel: w71 -> [w239] mode=indexing
            n114 = Equal?(x=w240, y=w239) -> (x = y?=w238:bool)
            n115 = case shown="True" w238 {
              tunnel: w237 -> [w241 _]
              tunnel: [w241 TRUE] -> w236
              frame False {
              }
              frame True {
              }
            }
          }
          n116 = case shown="True" w77 {
            tunnel: [w196 w199] -> w80
            tunnel: w71 -> [_ w197]
            tunnel: w76 -> [w196 _]
            frame False {
            }
            frame True {
              n117 = for {
                tunnel: w197 -> [w200] mode=indexing
                shift-right: [w201] -> w199
                shift-left: "" -> [w202]
                i -> [w203]
                n118 = case shown="0, Default" w203 {
                  tunnel: [w211 w213 w223 w231] -> w201
                  tunnel: w202 -> [w210 w214 w222 w228]
                  tunnel: w200 -> [w206 w215 w221 w229]
                  frame 0, Default {
                    n119 = Number To Fractional String(number=w206) -> (F-format string=w205:string)  [unwired: 3 in]
                    n120 = Concatenate Strings("Scan distance (µm): ", "\t", w205, "\t") -> (w207:string)
                    n121 = Concatenate Strings(w210, w207) -> (w211:string)
                  }
                  frame 1 {
                    n122 = Number To Fractional String(number=w215) -> (F-format string=w219:string)  [unwired: 3 in]
                    n123 = Concatenate Strings("Scan angle (degrees): ", "\t", w219, "\t") -> (w212:string)
                    n124 = Concatenate Strings(w214, w212) -> (w213:string)
                  }
                  frame 2 {
                    n125 = Number To Fractional String(number=w221) -> (F-format string=w227:string)  [unwired: 3 in]
                    n126 = Concatenate Strings("Record period (single track, s): ", "\t", w227, "\t") -> (w220:string)
                    n127 = Concatenate Strings(w222, w220) -> (w223:string)
                  }
                  frame 3 {
                    n128 = Number To Fractional String(number=w229) -> (F-format string=w235:string)  [unwired: 3 in]
                    n129 = Concatenate Strings("Time of movement (ms): ", "\t", w235, "\r\n") -> (w230:string)
                    n130 = Concatenate Strings(w228, w230) -> (w231:string)
                  }
                }
              }
            }
          }
          n131 = feedback #3() -> (w125:cluster{bool, bool})  [unwired: 1 in]
          n132 = case shown="True" w130 {
            tunnel: "VISA res. name" -> [_ w390]
            tunnel: [w386 w389] -> w120
            tunnel: "Manipulator Speed" -> [_ w389]
            tunnel: w135 -> [w386 _]
            tunnel: [w383 w388] -> w127
            tunnel: [w384 w387] -> w92
            tunnel: w125 -> [w385 _]
            frame False {
              n133 = Unbundle(w385) -> (w383:bool, w384:bool)
            }
            frame True {
              n134 = case shown="False" w389 {
                tunnel: w390 -> [w397 w458]
                tunnel: [FALSE w452] -> w387
                tunnel: [w391 FALSE] -> w388
                frame False {
                  n135 = stacked-sequence {
                    seq-local: [w398 _ _ _ _ _ _] -> [_ w408 _ _ _ _ _]
                    seq-local: [_ w404 _ _ _ _ _] -> [_ _ w417 _ _ _ _]
                    seq-local: [_ _ w411 _ _ _ _] -> [_ _ _ w420 _ _ _]
                    seq-local: [_ _ _ w421 _ _ _] -> [_ _ _ _ w432 _ _]
                    seq-local: [_ _ _ _ w431 _ _] -> [_ _ _ _ _ w437 _]
                    seq-local: [_ _ _ _ _ w436 _] -> [_ _ _ _ _ _ w448]
                    tunnel: w397 -> [w403 _ _ _ _ _ _]
                    tunnel: [_ _ w410 _ _ _ _] -> w395
                    tunnel: [_ _ _ _ w426 _ _] -> w393
                    tunnel: [_ _ _ _ _ _ w447] -> _
                    tunnel: [_ _ _ _ _ _ w442] -> w394
                    frame #0 {
                      w399 = u16 10 items=["1,0"=10, "1,5"=15, "2,0"=20] ("stop bits (10: 1 bit)")
                      n136 = call-poly "VISA Configure Serial Port"("VISA resource name"=w403, "baud rate (9600)"=u32 9600, "data bits (8)"=u16 8, "parity (0:none)"=enum16{"None", "Odd", "Even", "Mark", "Space"}."None", "stop bits (10: 1 bit)"=w399) -> ("VISA resource name out"=w398:refnum<visa-resource-name>)  [unwired: 9 in, 1 out]
                    }
                    frame #1 {
                      n137 = Wait (ms)(milliseconds to wait=u32 100) -> ()  [unwired: 1 out]
                      n138 = Concatenate Strings("ACC 10", "\r\n") -> (w405:string)
                      n139 = VISA Write(VISA resource name=w408, write buffer=w405) -> (VISA resource name out=w404:refnum<visa-resource-name>)  [unwired: 1 in, 2 out]
                    }
                    frame #2 {
                      n140 = property class="Instr"(reference=w417) -> (reference out=w418:refnum<visa-resource-name>, "Bytes at Port"=w416:u32)  [unwired: 1 in, 1 out]
                      n141 = Wait (ms)(milliseconds to wait=u32 100) -> ()  [unwired: 1 out]
                      n142 = VISA Read(VISA resource name=w418, byte count=w416) -> (VISA resource name out=w411:refnum<visa-resource-name>, read buffer=w415:string)  [unwired: 1 in, 2 out]
                      n143 = Concatenate Strings("A", "\r") -> (w412:string)
                      n144 = Equal?(x=w415, y=w412) -> (x = y?=w410:bool)
                    }
                    frame #3 {
                      n145 = Wait (ms)(milliseconds to wait=u32 100) -> ()  [unwired: 1 out]
                      n146 = Concatenate Strings("FIRST 1000", "\r\n") -> (w422:string)
                      n147 = VISA Write(VISA resource name=w420, write buffer=w422) -> (VISA resource name out=w421:refnum<visa-resource-name>)  [unwired: 1 in, 2 out]
                    }
                    frame #4 {
                      n148 = property class="Instr"(reference=w432) -> (reference out=w433:refnum<visa-resource-name>, "Bytes at Port"=w434:u32)  [unwired: 1 in, 1 out]
                      n149 = Wait (ms)(milliseconds to wait=u32 100) -> ()  [unwired: 1 out]
                      n150 = Concatenate Strings("A", "\r") -> (w427:string)
                      n151 = VISA Read(VISA resource name=w433, byte count=w434) -> (VISA resource name out=w431:refnum<visa-resource-name>, read buffer=w430:string)  [unwired: 1 in, 2 out]
                      n152 = Equal?(x=w430, y=w427) -> (x = y?=w426:bool)
                    }
                    frame #5 {
                      n153 = Wait (ms)(milliseconds to wait=u32 100) -> ()  [unwired: 1 out]
                      n154 = Concatenate Strings("TOP 1000", "\r\n") -> (w438:string)
                      n155 = VISA Write(VISA resource name=w437, write buffer=w438) -> (VISA resource name out=w436:refnum<visa-resource-name>)  [unwired: 1 in, 2 out]
                    }
                    frame #6 {
                      n156 = property class="Instr"(reference=w448) -> (reference out=w449:refnum<visa-resource-name>, "Bytes at Port"=w450:u32)  [unwired: 1 in, 1 out]
                      n157 = Wait (ms)(milliseconds to wait=u32 100) -> ()  [unwired: 1 out]
                      n158 = VISA Read(VISA resource name=w449, byte count=w450) -> (VISA resource name out=w447:refnum<visa-resource-name>, read buffer=w443:string)  [unwired: 1 in, 2 out]
                      n159 = Concatenate Strings("A", "\r") -> (w446:string)
                      n160 = Equal?(x=w443, y=w446) -> (x = y?=w442:bool)
                    }
                  }
                  n161 = And(x=w395, y=w394) -> (x .and. y?=w396:bool)
                  n162 = And(x=w396, y=w393) -> (x .and. y?=w391:bool)
                }
                frame True {
                  n163 = stacked-sequence {
                    seq-local: [w459 _ _ _ _ _ _] -> [_ w469 _ _ _ _ _]
                    seq-local: [_ w465 _ _ _ _ _] -> [_ _ w478 _ _ _ _]
                    seq-local: [_ _ w472 _ _ _ _] -> [_ _ _ w481 _ _ _]
                    seq-local: [_ _ _ w482 _ _ _] -> [_ _ _ _ w493 _ _]
                    seq-local: [_ _ _ _ w492 _ _] -> [_ _ _ _ _ w498 _]
                    seq-local: [_ _ _ _ _ w497 _] -> [_ _ _ _ _ _ w509]
                    tunnel: w458 -> [w464 _ _ _ _ _ _]
                    tunnel: [_ _ w471 _ _ _ _] -> w456
                    tunnel: [_ _ _ _ w487 _ _] -> w454
                    tunnel: [_ _ _ _ _ _ w508] -> _
                    tunnel: [_ _ _ _ _ _ w503] -> w455
                    frame #0 {
                      w460 = u16 10 items=["1,0"=10, "1,5"=15, "2,0"=20] ("stop bits (10: 1 bit)")
                      n164 = call-poly "VISA Configure Serial Port"("VISA resource name"=w464, "baud rate (9600)"=u32 9600, "data bits (8)"=u16 8, "parity (0:none)"=enum16{"None", "Odd", "Even", "Mark", "Space"}."None", "stop bits (10: 1 bit)"=w460) -> ("VISA resource name out"=w459:refnum<visa-resource-name>)  [unwired: 9 in, 1 out]
                    }
                    frame #1 {
                      n165 = Wait (ms)(milliseconds to wait=u32 100) -> ()  [unwired: 1 out]
                      n166 = Concatenate Strings("ACC 500", "\r\n") -> (w466:string)
                      n167 = VISA Write(VISA resource name=w469, write buffer=w466) -> (VISA resource name out=w465:refnum<visa-resource-name>)  [unwired: 1 in, 2 out]
                    }
                    frame #2 {
                      n168 = property class="Instr"(reference=w478) -> (reference out=w479:refnum<visa-resource-name>, "Bytes at Port"=w477:u32)  [unwired: 1 in, 1 out]
                      n169 = Wait (ms)(milliseconds to wait=u32 100) -> ()  [unwired: 1 out]
                      n170 = VISA Read(VISA resource name=w479, byte count=w477) -> (VISA resource name out=w472:refnum<visa-resource-name>, read buffer=w476:string)  [unwired: 1 in, 2 out]
                      n171 = Concatenate Strings("A", "\r") -> (w473:string)
                      n172 = Equal?(x=w476, y=w473) -> (x = y?=w471:bool)
                    }
                    frame #3 {
                      n173 = Wait (ms)(milliseconds to wait=u32 100) -> ()  [unwired: 1 out]
                      n174 = Concatenate Strings("FIRST 1000", "\r\n") -> (w483:string)
                      n175 = VISA Write(VISA resource name=w481, write buffer=w483) -> (VISA resource name out=w482:refnum<visa-resource-name>)  [unwired: 1 in, 2 out]
                    }
                    frame #4 {
                      n176 = property class="Instr"(reference=w493) -> (reference out=w494:refnum<visa-resource-name>, "Bytes at Port"=w495:u32)  [unwired: 1 in, 1 out]
                      n177 = Wait (ms)(milliseconds to wait=u32 100) -> ()  [unwired: 1 out]
                      n178 = Concatenate Strings("A", "\r") -> (w488:string)
                      n179 = VISA Read(VISA resource name=w494, byte count=w495) -> (VISA resource name out=w492:refnum<visa-resource-name>, read buffer=w491:string)  [unwired: 1 in, 2 out]
                      n180 = Equal?(x=w491, y=w488) -> (x = y?=w487:bool)
                    }
                    frame #5 {
                      n181 = Wait (ms)(milliseconds to wait=u32 100) -> ()  [unwired: 1 out]
                      n182 = Concatenate Strings("TOP 30000", "\r\n") -> (w499:string)
                      n183 = VISA Write(VISA resource name=w498, write buffer=w499) -> (VISA resource name out=w497:refnum<visa-resource-name>)  [unwired: 1 in, 2 out]
                    }
                    frame #6 {
                      n184 = property class="Instr"(reference=w509) -> (reference out=w510:refnum<visa-resource-name>, "Bytes at Port"=w511:u32)  [unwired: 1 in, 1 out]
                      n185 = Wait (ms)(milliseconds to wait=u32 100) -> ()  [unwired: 1 out]
                      n186 = VISA Read(VISA resource name=w510, byte count=w511) -> (VISA resource name out=w508:refnum<visa-resource-name>, read buffer=w504:string)  [unwired: 1 in, 2 out]
                      n187 = Concatenate Strings("A", "\r") -> (w507:string)
                      n188 = Equal?(x=w504, y=w507) -> (x = y?=w503:bool)
                    }
                  }
                  n189 = And(x=w456, y=w455) -> (x .and. y?=w457:bool)
                  n190 = And(x=w457, y=w454) -> (x .and. y?=w452:bool)
                }
              }
            }
          }
          "fast" <- w92
          n191 = Bundle(w127, w92) -> (w126:cluster{bool, bool})  [unwired: 1 in]
          n192 = feedback-in #3(w126) -> ()
          n193 = Build Array(w128, w127, w70, w121) -> (w91:bool[])
          n194 = for {
            N: 4 -> [_]
            tunnel: w91 -> [w343] mode=indexing
            shift-right: [w341] -> w93
            shift-left: 0 -> [w342]
            n195 = case shown="False" w343 {
              tunnel: w342 -> [w344 w347]
              tunnel: [w344 w345] -> w341
              frame False {
              }
              frame True {
                n196 = Add(x=w347, y=1) -> (x+y=w345:i32)
              }
            }
          }
          n197 = Index Array(array=w91, index=0 ("Index")) -> (element=→"Ind. Channel Out":bool)
          n198 = Index Array(array=w91, index=1 ("Index")) -> (element=→"slow":bool)
          n199 = Equal?(x=w93, y=4) -> (x = y?=w160:bool)
          n200 = Index Array(array=w91, index=2 ("Index")) -> (element=→"Ind. Channel In":bool)
          n201 = Index Array(array=w91, index=3 ("Index")) -> (element=→"Data File":bool)
          n202 = And(x=w90, y=w160) -> (x .and. y?=w84:bool)
          n203 = Bundle("Data file"=w116) -> (w169:cluster{"Data file ":path})  [unwired: 1 in]
          "Output SISE ch 2" <- "SISE channel 2"
          "SISE channel 1" <- w110
          "Output V ch 1" <- "V channel 1"
          "Output V ch 2" <- "V channel 2"
          "right" <- "Position of manipulator"
        }
        n204 = Unbundle(w51) -> ("refnum out"=w46:refnum<file>, "status"=w50:bool, "code"=w49:i32, "source"=w48:string)
        n205 = Bundle("status"=w50, "code"=w49, "source"=w48) -> (w47:errorcluster)  [unwired: 1 in]
        n206 = Concatenate Strings(w35, w36) -> (w34:string)
        n207 = Write to Text File(file (use dialog)=w46, text=w34, error in=w47) -> (refnum out=w44:refnum<file>, error out=w45:errorcluster)  [unwired: 1 in, 1 out]
        n208 = Unbundle(w45) -> ("status"=w43:bool, "code"=w42:i32, "source"=w41:string)
        n209 = Bundle("refnum out"=w44, "status"=w43, "code"=w42, "source"=w41) -> (w40:T4)  [unwired: 1 in]
      }
      frame 1 {
        # "Total number of \nmeasueremnt cycles"
        n210 = Index Array(array=w544, index=2 ("Index")) -> (element=w540:dbl)
        n211 = Build Array(0.0, 0.0, 0.0, 0.0, 0.0) -> (w521:dbl[])
        n212 = Multiply(x=w540, y=300.0 ("x")) -> (x*y=w545:dbl)
        n213 = Get Date/Time In Seconds() -> (seconds since 1Jan1904=w563:timestamp)
        n214 = Bundle(string[] [], dbl[][] []) -> (w537:cluster{string[], dbl[][]})  [unwired: 1 in]
        n215 = Build Array(0.0 ("Element"), 0.0 ("Element"), 0.0 ("Element")) -> (w558:dbl[])
        n216 = for {
          N: w545 -> [_]
          shift-right: [w567] -> w541
          shift-left: dbl[][] [] -> [w566]
          tunnel: w521 -> [w565]
          n217 = Insert Into Array(array=w566, new element=w565) -> (w567:dbl[][])  [unwired: 2 in]
        }
        n218 = Obtain Queue(element data type=w537) -> (queue out=w547:refnum<queue>, error out=w550:errorcluster)  [unwired: 4 in, 1 out]
        n219 = while {
          tunnel: w544 -> [w1090]
          tunnel: w563 -> [w1063]
          tunnel: w557 -> [w1101]
          shift-right: [w1100] -> _
          shift-left: "P0: P1:" -> [w1103]
          shift-right: [w1099] -> _
          shift-left: w558 -> [w1102]
          tunnel: [w1098] -> w556
          tunnel: w555 -> [w1097]
          tunnel: [w1092] -> w518
          tunnel: [w1091] -> w517
          shift-right: [w1085] -> w549
          shift-left: w547 -> [w1083]
          shift-right: [w1084] -> w548
          shift-left: w550 -> [w1088]
          tunnel: w534 -> [w1080]
          tunnel: [w1074] -> w516
          tunnel: [w1073] -> w515
          shift-right: [w1069] -> _
          shift-left: "" -> [w1071]
          tunnel: string[] [] -> [w1072]
          tunnel: [w1070] -> _
          tunnel: w513 -> [w1066]
          tunnel: [w1065] -> w527
          shift-right: [w1062] -> _
          shift-left: 0 -> [w1061]
          tunnel: w513 -> [w1060]
          i -> [w1068]
          stop <- w1064 stop-if-true
          n220 = Unbundle(w1097) -> ("task out"=w1067:refnum<k21>, "status"=w1096:bool, "code"=w1095:i32, "source"=w1094:string)
          n221 = Unbundle(w1080) -> ("refnum out"=w1076:refnum<file>, "status"=w1079:bool, "code"=w1077:i32, "source"=w1078:string)
          n222 = Divide(x=w1068, y=2) -> (x/y=w1106:dbl)
          n223 = Round Toward -Infinity(1:w1106) -> (0:w1107:dbl)
          n224 = Bundle("status"=w1096, "code"=w1095, "source"=w1094) -> (w1093:errorcluster)  [unwired: 1 in]
          n225 = Bundle("status"=w1079, "code"=w1077, "source"=w1078) -> (w1075:errorcluster)  [unwired: 1 in]
          n226 = Equal?(x=w1106, y=w1107) -> (x = y?=w1104:bool)
          n227 = while {
            tunnel: w1090 -> [w1228]
            shift-right: [w1144] -> w1064
            shift-left: FALSE -> [w1224]
            tunnel: w1104 -> [w1158]
            tunnel: w1068 -> [w1213]
            tunnel: w1090 -> [w1171]
            tunnel: w1090 -> [w1206]
            tunnel: w1101 -> [w1205]
            shift-right: [w1145] -> w1100
            shift-left: w1103 -> [w1208]
            shift-right: [w1204] -> w1099
            shift-left: w1102 -> [w1207]
            tunnel: [w1203] -> w1098
            tunnel: w1068 -> [w1195]
            tunnel: w1093 -> [w1193]
            tunnel: w1067 -> [w1194]
            tunnel: [w1164] -> w1092
            tunnel: [w1192] -> w1091
            tunnel: w1090 -> [w1163]
            shift-right: [w1161] -> w1082
            shift-left: dbl[][] [] -> [w1156]
            tunnel: [w1187] -> w1087
            tunnel: [w1186] -> w1086
            tunnel: w1083 -> [w1187]
            tunnel: w1088 -> [w1186]
            tunnel: w1068 -> [w1184]
            tunnel: w1076 -> [w1178]
            tunnel: w1075 -> [w1179]
            tunnel: [w1177] -> w1073
            tunnel: [w1176] -> w1074
            shift-right: [w1173] -> w1070
            shift-left: w1072 -> [w1181]
            shift-right: [w1172] -> w1069
            shift-left: w1071 -> [w1188]
            tunnel: w1068 -> [w1170]
            tunnel: w1066 -> [w1155]
            tunnel: w1066 -> [w1159]
            tunnel: [w1155] -> w1065
            tunnel: w1063 -> [w1123]
            shift-right: [w1119] -> w1062
            shift-left: w1061 -> [w1129]
            tunnel: w1060 -> [w1126]
            i -> [w1114]
            stop <- w1226 stop-if-true
            w1131 = 0 ("Index")
            # "Stop measurement cycle"
            # "Number of measurement loops"
            # "Measurement time (ms)"
            # "Control timing"
            # "Write to file"
            # "Add position / Event marks"
            # "Feed graphs"
            # "Get voltage data"
            # "Get time (s) / calculate position of probe"
            # "Control manipulator"
            # "Set graphs and controls"
            # "Set # of cycles"
            # "Stop experiment"
            n228 = Get Date/Time In Seconds() -> (seconds since 1Jan1904=w1223:timestamp)
            n229 = Equal To 0?(x=w1114) -> (x = 0?=w1189:bool)
            n230 = Greater Or Equal?(x=w1184, y=2) -> (x >= y?=w1183:bool)
            "E-mark on" <- w1183
            n231 = Subtract(x=w1223, y=w1123) -> (x-y=w1121:dbl)
            n232 = call-poly <vilib>:"DAQmx Read.vi"("task/channels in"=w1194, "error in"=w1193) -> ("task out"=w1164:refnum<k21>, "data"=w1130:dbl[][], "error out"=w1192:errorcluster)  [unwired: 11 in]
            n233 = Add(x=w1129, y=1) -> (x+y=w1119:i32)
            n234 = Index Array(array=w1171, index=2) -> (element=w1211:dbl)
            n235 = Equal?(x=w1170, y=0) -> (x = y?=w1167:bool)
            n236 = Equal?(x=w1114, y=0) -> (x = y?=w1166:bool)
            n237 = Multiply(x=w1211, y=100.0) -> (x*y=w1210:dbl)
            n238 = Multiply(x=w1119, y=10) -> (x*y=w1116:i32)
            n239 = Multiply(x=w1121, y=1000.0) -> (x*y=w1109:dbl)
            n240 = Index Array(array=w1228, index=2) -> (element=w1231:dbl)
            n241 = case shown="True" w1183 {
              tunnel: [FALSE "Add Mark"] -> w1182
              tunnel: w1181 -> [_ w1308]
              frame False {
              }
              frame True {
                n242 = Array Size(array=w1308) -> (size(s)=w1312:i32)
                n243 = Subtract(x=w1312, y=1) -> (x-y=w1310:i32)
                n244 = Index Array(array=w1308, index=w1310) -> (element=→"String":string)
              }
            }
            n245 = Index Array(array=w1130, index (row)=w1131, index (col)=w1131) -> (element=w1139:dbl)
            n246 = Index Array(array=w1130, index (row)=1 ("Index"), index (col)=w1131) -> (element=w1138:dbl)
            n247 = Index Array(array=w1130, index (row)=2 ("Index"), index (col)=w1131) -> (element=w1136:dbl)
            n248 = Index Array(array=w1130, index (row)=3 ("Index"), index (col)=w1131) -> (element=w1137:dbl)
            n249 = And(x=w1167, y=w1166) -> (x .and. y?=w1165:bool)
            n250 = call "Feed-Position-Graph (SubVI).vi"("Array 2"=w1163, "Array"=w1156) -> ("Array 3"=→"Position probe":cluster{dbl[], dbl[]}[])  [unwired: 9 in]
            n251 = Subtract(x=w1109, y=w1116) -> (x-y=w1118:dbl)
            n252 = Subtract(x=w1210, y=10.0) -> (x-y=w1220:dbl)
            n253 = Subtract(x=w1210, y=20.0) -> (x-y=w1219:dbl)
            n254 = Multiply(x=w1231, y=100.0) -> (x*y=w1216:dbl)
            n255 = Index Array(array=w1126, index=4) -> (element=w1125:bool)
            n256 = Multiply(x=w1118, y=-1.0) -> (x*y=w1113:dbl)
            n257 = Equal?(x=w1213, y=0) -> (x = y?=w1151:bool)
            n258 = Build Array(0, 10, w1219, w1220) -> (w1115:dbl[])
            n259 = Divide(x=w1139, y=-0.0333) -> (x/y=w1134:dbl)
            n260 = Divide(x=w1138, y=-0.0333) -> (x/y=w1135:dbl)
            n261 = Add(x=1 ("y"), y=w1114) -> (x+y=w1227:i32)
            n262 = case shown="True" w1151 {
              tunnel: [w1411 w1429] -> w1150
              tunnel: w1115 -> [w1410 w1428]
              tunnel: w1114 -> [w1409 w1427]
              frame False {
                n263 = for {
                  tunnel: w1410 -> [w1418] mode=indexing
                  tunnel: w1409 -> [w1419]
                  shift-right: [w1416] -> w1411
                  shift-left: 0 -> [w1417]
                  i -> [w1414]
                  n264 = Equal?(x=w1418, y=w1419) -> (x = y?=w1415:bool)
                  n265 = case shown="True" w1415 {
                    tunnel: w1414 -> [_ w1422]
                    tunnel: [0 w1421] -> w1413
                    frame False {
                    }
                    frame True {
                      n266 = case shown="3" w1422 {
                        tunnel: [1 2 3 5] -> w1421
                        frame 0, Default {
                        }
                        frame 1 {
                        }
                        frame 2 {
                        }
                        frame 3 {
                        }
                      }
                    }
                  }
                  n267 = Add(x=w1417, y=w1413) -> (x+y=w1416:i32)
                }
              }
              frame True {
                n268 = for {
                  tunnel: w1428 -> [w1436] mode=indexing
                  tunnel: w1427 -> [w1437]
                  shift-right: [w1434] -> w1429
                  shift-left: 0 -> [w1435]
                  i -> [w1433]
                  n269 = Equal?(x=w1436, y=w1437) -> (x = y?=w1431:bool)
                  n270 = case shown="True" w1431 {
                    tunnel: w1433 -> [_ w1439]
                    tunnel: [0 w1440] -> w1432
                    frame False {
                    }
                    frame True {
                      n271 = case shown="0, Default" w1439 {
                        tunnel: [0 0 3 4] -> w1440
                        frame 0, Default {
                        }
                        frame 1 {
                        }
                        frame 2 {
                        }
                        frame 3 {
                        }
                      }
                    }
                  }
                  n272 = Add(x=w1435, y=w1432) -> (x+y=w1434:i32)
                }
              }
            }
            n273 = Build Array(w1134, w1135, w1136, w1137) -> (w1133:dbl[])
            n274 = Equal?(x=w1216, y=w1227) -> (x = y?=w1226:bool)
            n275 = for {
              tunnel: w1133 -> [w1285] mode=indexing
              tunnel: w1155 -> [w1288] mode=indexing
              shift-right: [w1286] -> w1154
              shift-left: dbl[] [] -> [w1287]
              shift-right: [w1283] -> w1147
              shift-left: dbl[] [] -> [w1284]
              n276 = case shown="False" w1288 {
                tunnel: w1287 -> [w1292 w1297]
                tunnel: [w1292 w1296] -> w1286
                tunnel: w1285 -> [_ w1293]
                tunnel: w1284 -> [w1291 w1295]
                tunnel: [w1290 w1294] -> w1283
                frame False {
                  n277 = Insert Into Array(array=w1291, new element=0.0 ("Neues Element/Teil-Array")) -> (w1290:dbl[])  [unwired: 1 in]
                }
                frame True {
                  n278 = Insert Into Array(array=w1297, new element=w1293) -> (w1296:dbl[])  [unwired: 1 in]
                  n279 = Insert Into Array(array=w1295, new element=w1293) -> (w1294:dbl[])  [unwired: 1 in]
                }
              }
            }
            n280 = Index Array(array=w1171, index=3 ("Index")) -> (element=w1201:dbl)
            n281 = Index Array(array=w1171, index=0 ("Index")) -> (element=w1197:dbl)
            n282 = case shown="\"SISE chan #1\", Default" "?" {
              selector: "?" -> [w1252 w1262 w1270 w1278]
              tunnel: w1163 -> [w1257 w1264 w1274 w1281]
              tunnel: w1156 -> [w1258 w1265 w1273 w1282]
              tunnel: w1159 -> [w1254 w1261 w1268 w1277]
              tunnel: "Start fit (% of rec. period)" -> [w1256 w1263 w1272 w1280]
              frame "SISE chan #1", Default {
                n283 = Index Array(array=w1254, index=w1252) -> (element=w1253:bool)
                n284 = call "Feed-SISE-Probe-Graph.vi"("Boolesch"=w1253, "Numerisch"=2, "Array 2"=w1258, "Array"=w1257, "Start fit (% of rec. period)"=w1256) -> ("Array 3"=→"Vprobe SISE 1":cluster{dbl[], dbl[]}[])  [unwired: 6 in]
              }
              frame "SISE chan #2" {
                n285 = Index Array(array=w1261, index=w1262) -> (element=w1260:bool)
                n286 = call "Feed-SISE-Probe-Graph.vi"("Boolesch"=w1260, "Numerisch"=3, "Array 2"=w1265, "Array"=w1264, "Start fit (% of rec. period)"=w1263) -> ("Array 3"=→"Vprobe SISE 2":cluster{dbl[], dbl[]}[])  [unwired: 6 in]
              }
              frame "V chan #1" {
                n287 = Index Array(array=w1268, index=w1270) -> (element=w1269:bool)
                n288 = call "Feed-V-Probe-Graph.vi"("Boolesch"=w1269, "Numerisch"=4, "Array 2"=w1273, "Array"=w1274, "Start fit (% of rec. period)"=w1272) -> ("Array 3"=→"Vprobe V 1":cluster{dbl[], dbl[]}[])  [unwired: 6 in]
              }
              frame "V chan #2" {
                n289 = Index Array(array=w1277, index=w1278) -> (element=w1276:bool)
                n290 = call "Feed-V-Probe-Graph.vi"("Boolesch"=w1276, "Numerisch"=5, "Array 2"=w1282, "Array"=w1281, "Start fit (% of rec. period)"=w1280) -> ("Array 3"=→"Vprobe V 2":cluster{dbl[], dbl[]}[])  [unwired: 6 in]
              }
            }
            n291 = Divide(x=w1201, y=10.0) -> (x/y=w1196:dbl)
            n292 = for {
              tunnel: w1115 -> [w1235] mode=indexing
              tunnel: w1114 -> [w1236]
              shift-right: [w1232] -> w1110
              shift-left: FALSE -> [w1233]
              n293 = Equal?(x=w1235, y=w1236) -> (x = y?=w1234:bool)
              n294 = case shown="False" w1234 {
                tunnel: w1233 -> [w1237 _]
                tunnel: [w1237 TRUE] -> w1232
                frame False {
                }
                frame True {
                }
              }
            }
            n295 = case shown="1" w1150 {
              tunnel: w1205 -> [w1445 w1458 w1502 w1509 w1521 w1568]
              tunnel: w1207 -> [w1447 w1465 w1505 w1508 w1520 w1567]
              tunnel: [w1447 w1465 w1505 w1508 w1519 w1566] -> w1204
              tunnel: w1206 -> [_ w1464 _ _ _ _]
              tunnel: w1158 -> [_ w1453 _ _ w1513 w1560]
              tunnel: w1208 -> [w1446 w1452 w1501 w1507 w1516 w1563]
              tunnel: [w1446 w1452 w1501 w1507 w1517 w1564] -> w1145
              tunnel: [w1445 w1451 w1500 w1506 w1514 w1561] -> w1203
              tunnel: w1125 -> [_ w1448 _ _ _ _]
              frame 0, Default {
              }
              frame 1 {
                n296 = Index Array(array=w1464, index=0) -> (element=w1466:dbl)
                n297 = Index Array(array=w1464, index=1) -> (element=w1457:dbl)
                n298 = case shown="True" w1448 {
                  tunnel: [-10.0 10.0] -> w1449
                  frame False {
                  }
                  frame True {
                  }
                }
                n299 = Cosine(x=w1457) -> (cos(x)=w1456:dbl)
                n300 = Sine(x=w1457) -> (sin(x)=w1455:dbl)
                n301 = Multiply(x=w1466, y=w1456) -> (x*y=w1463:dbl)
                n302 = Multiply(x=w1466, y=w1455) -> (x*y=w1462:dbl)
                n303 = Multiply(x=w1462, y=10.0) -> (x*y=w1461:dbl)
                n304 = Multiply(x=w1463, y=w1449) -> (x*y=w1460:dbl)
                n305 = for {
                  tunnel: w1465 -> [w1480] mode=indexing
                  tunnel: w1460 -> [w1482]
                  tunnel: w1461 -> [w1481]
                  shift-right: [w1476] -> w1454
                  shift-left: "ABS " -> [w1478]
                  tunnel: w1453 -> [w1471]
                  i -> [w1473]
                  n306 = case shown="False" w1471 {
                    tunnel: w1473 -> [w1483 _]
                    tunnel: [w1483 1] -> w1472
                    frame False {
                    }
                    frame True {
                    }
                  }
                  n307 = case shown="0, Default" w1472 {
                    tunnel: w1482 -> [w1494 _ _]
                    tunnel: w1481 -> [_ _ w1498]
                    tunnel: w1480 -> [w1495 w1496 w1499]
                    tunnel: [w1493 w1496 w1497] -> w1479
                    frame 0, Default {
                      n308 = Add(x=w1495, y=w1494) -> (x+y=w1493:dbl)
                    }
                    frame 1 {
                    }
                    frame 2 {
                      n309 = Add(x=w1499, y=w1498) -> (x+y=w1497:dbl)
                    }
                  }
                  n310 = Number To Decimal String(number=w1479) -> (decimal integer string=w1477:string)  [unwired: 1 in]
                  n311 = Equal?(x=2, y=w1473) -> (x = y?=w1474:bool)
                  n312 = case shown="True" w1474 {
                    tunnel: w1478 -> [w1488 w1492]
                    tunnel: w1477 -> [w1487 w1490]
                    tunnel: [w1485 w1491] -> w1476
                    frame False {
                      n313 = Concatenate Strings(w1488, w1487, "\t") -> (w1485:string)
                    }
                    frame True {
                      n314 = Concatenate Strings(w1492, w1490, "\r\n") -> (w1491:string)
                    }
                  }
                }
                n315 = VISA Write(VISA resource name=w1458, write buffer=w1454) -> (VISA resource name out=w1451:refnum<visa-resource-name>)  [unwired: 1 in, 2 out]
              }
              frame 2 {
                n316 = property class="Instr"(reference=w1502) -> (reference out=w1503:refnum<visa-resource-name>, "Bytes at Port"=w1504:u32)  [unwired: 1 in, 1 out]
                n317 = VISA Read(VISA resource name=w1503, byte count=w1504) -> (VISA resource name out=w1500:refnum<visa-resource-name>)  [unwired: 1 in, 3 out]
              }
              frame 3 {
                n318 = Concatenate Strings("POS", "\r\n") -> (w1512:string)
                n319 = VISA Write(VISA resource name=w1509, write buffer=w1512) -> (VISA resource name out=w1506:refnum<visa-resource-name>)  [unwired: 1 in, 2 out]
              }
              frame 4 {
                n320 = property class="Instr"(reference=w1521) -> (reference out=w1523:refnum<visa-resource-name>, "Bytes at Port"=w1522:u32)  [unwired: 1 in, 1 out]
                n321 = VISA Read(VISA resource name=w1523, byte count=w1522) -> (VISA resource name out=w1515:refnum<visa-resource-name>, read buffer=w1518:string)  [unwired: 1 in, 2 out]
                n322 = case shown="True" w1513 {
                  tunnel: w1520 -> [w1539 w1558]
                  tunnel: [w1539 w1557] -> w1519
                  tunnel: w1518 -> [w1528 w1543]
                  tunnel: [w1533 w1552] -> w1517
                  tunnel: w1516 -> [w1532 w1551]
                  tunnel: w1515 -> [w1524 w1542]
                  tunnel: [w1524 w1542] -> w1514
                  frame False {
                    n323 = Match Pattern(string=w1532, regular expression="P0:") -> (match substring=w1537:string, after substring=w1536:string)  [unwired: 1 in, 2 out]
                    n324 = String Length(string=w1528) -> (length=w1531:i32)
                    n325 = Match Pattern(string=w1536, regular expression="P1:") -> (before substring=w1525:string, match substring=w1538:string)  [unwired: 1 in, 2 out]
                    n326 = Subtract(x=w1531, y=1) -> (x-y=w1529:i32)
                    n327 = String Subset(string=w1528, length (rest)=w1529) -> (substring=w1527:string)  [unwired: 1 in]
                    n328 = Concatenate Strings(w1537, w1525, w1538, w1527, "\t") -> (w1533:string)
                  }
                  frame True {
                    n329 = Match Pattern(string=w1551, regular expression="P0:") -> (match substring=w1553:string, after substring=w1555:string)  [unwired: 1 in, 2 out]
                    n330 = String Length(string=w1543) -> (length=w1550:i32)
                    n331 = Subtract(x=w1550, y=1) -> (x-y=w1548:i32)
                    n332 = Match Pattern(string=w1555, regular expression="P1:") -> (match substring=w1545:string, after substring=w1546:string)  [unwired: 1 in, 2 out]
                    n333 = String Subset(string=w1543, length (rest)=w1548) -> (substring=w1547:string)  [unwired: 1 in]
                    n334 = Concatenate Strings(w1553, w1547, "\t", w1545, w1546) -> (w1552:string)
                    n335 = call "GetAxisValuesI (SubVI).vi"("read buffer"=w1543) -> ("Array"=w1540:dbl[])  [unwired: 10 in]
                    n336 = Replace Array Subset(array=w1558, new element=w1540, index=0 ("Index")) -> (w1557:dbl[])
                  }
                }
              }
              frame 5 {
                n337 = property class="Instr"(reference=w1568) -> (reference out=w1570:refnum<visa-resource-name>, "Bytes at Port"=w1569:u32)  [unwired: 1 in, 1 out]
                n338 = VISA Read(VISA resource name=w1570, byte count=w1569) -> (VISA resource name out=w1562:refnum<visa-resource-name>, read buffer=w1565:string)  [unwired: 1 in, 2 out]
                n339 = case shown="True" w1560 {
                  tunnel: w1567 -> [w1586 w1605]
                  tunnel: [w1586 w1604] -> w1566
                  tunnel: w1565 -> [w1575 w1590]
                  tunnel: [w1580 w1599] -> w1564
                  tunnel: w1563 -> [w1579 w1598]
                  tunnel: w1562 -> [w1571 w1588]
                  tunnel: [w1571 w1587] -> w1561
                  tunnel: "Enable change position 0" -> [_ w1589]
                  frame False {
                    n340 = Match Pattern(string=w1579, regular expression="P0:") -> (match substring=w1584:string, after substring=w1583:string)  [unwired: 1 in, 2 out]
                    n341 = String Length(string=w1575) -> (length=w1578:i32)
                    n342 = Match Pattern(string=w1583, regular expression="P1:") -> (before substring=w1572:string, match substring=w1585:string)  [unwired: 1 in, 2 out]
                    n343 = Subtract(x=w1578, y=1) -> (x-y=w1576:i32)
                    n344 = String Subset(string=w1575, length (rest)=w1576) -> (substring=w1574:string)  [unwired: 1 in]
                    n345 = Concatenate Strings(w1584, w1572, w1585, w1574, "\t") -> (w1580:string)
                  }
                  frame True {
                    n346 = Match Pattern(string=w1598, regular expression="P0:") -> (match substring=w1600:string, after substring=w1602:string)  [unwired: 1 in, 2 out]
                    n347 = String Length(string=w1590) -> (length=w1597:i32)
                    n348 = Subtract(x=w1597, y=1) -> (x-y=w1595:i32)
                    n349 = Match Pattern(string=w1602, regular expression="P1:") -> (match substring=w1592:string, after substring=w1593:string)  [unwired: 1 in, 2 out]
                    n350 = String Subset(string=w1590, length (rest)=w1595) -> (substring=w1594:string)  [unwired: 1 in]
                    n351 = case shown="True" w1589 {
                      tunnel: w1605 -> [w1607 w1613]
                      tunnel: [w1607 w1612] -> w1604
                      tunnel: w1590 -> [_ w1611]
                      tunnel: w1588 -> [w1606 w1608]
                      tunnel: [w1606 w1608] -> w1587
                      frame False {
                      }
                      frame True {
                        n352 = call "GetAxisValuesI (SubVI).vi"("read buffer"=w1611) -> ("Array"=w1609:dbl[])  [unwired: 10 in]
                        n353 = Replace Array Subset(array=w1613, new element=w1609, index=0 ("Index")) -> (w1612:dbl[])
                      }
                    }
                    n354 = Concatenate Strings(w1600, w1594, "\t", w1592, w1593) -> (w1599:string)
                  }
                }
              }
            }
            n355 = case shown="True" w1189 {
              tunnel: w1145 -> [_ w1335]
              tunnel: [w1318 w1335] -> w1174
              tunnel: w1182 -> [w1319 _]
              tunnel: w1181 -> [w1314 w1343]
              tunnel: w1121 -> [w1317 w1342]
              tunnel: [w1316 w1335] -> w1172
              tunnel: w1188 -> [w1316 w1336]
              tunnel: [w1315 w1341] -> w1173
              frame False {
                n356 = case shown="True" w1319 {
                  tunnel: ["" "Event Mark"] -> w1318
                  tunnel: w1317 -> [_ w1333]
                  tunnel: w1314 -> [w1321 w1326]
                  tunnel: [w1321 w1327] -> w1315
                  frame False {
                  }
                  frame True {
                    n357 = Divide(x=w1333, y=60.0) -> (x/y=w1331:dbl)
                    n358 = Number To Fractional String(number=w1331, precision (6)=i16 2 ("Genauigkeit (6)")) -> (F-format string=w1329:string)  [unwired: 2 in]
                    n359 = Concatenate Strings(w1329, " min: ", "\t", "Event Mark", "\t") -> (w1325:string)
                    n360 = Insert Into Array(array=w1326, new element=w1325) -> (w1327:string[])  [unwired: 1 in]
                  }
                }
              }
              frame True {
                n361 = Match Pattern(string=w1335, regular expression="P1:") -> (before substring=w1339:string)  [unwired: 1 in, 3 out]
                n362 = Match Pattern(string=w1336, regular expression="P1:") -> (before substring=w1337:string)  [unwired: 1 in, 3 out]
                n363 = Not Equal?(x=w1339, y=w1337) -> (x != y?=w1334:bool)
                n364 = case shown="True" w1334 {
                  tunnel: w1343 -> [w1344 w1366]
                  tunnel: [w1344 w1367] -> w1341
                  tunnel: w1335 -> [_ w1355]
                  tunnel: w1336 -> [_ w1354]
                  tunnel: w1342 -> [_ w1352]
                  frame False {
                  }
                  frame True {
                    n365 = Divide(x=w1352, y=60.0) -> (x/y=w1350:dbl)
                    n366 = Match Pattern(string=w1355, regular expression="P0:") -> (after substring=w1365:string)  [unwired: 1 in, 3 out]
                    n367 = Number To Fractional String(number=w1350, precision (6)=i16 2) -> (F-format string=w1346:string)  [unwired: 2 in]
                    n368 = Match Pattern(string=w1354, regular expression="P0:") -> (after substring=w1360:string)  [unwired: 1 in, 3 out]
                    n369 = Match Pattern(string=w1365, regular expression="P1:") -> (before substring=w1364:string)  [unwired: 1 in, 3 out]
                    n370 = Match Pattern(string=w1360, regular expression="P1:") -> (before substring=w1359:string)  [unwired: 1 in, 3 out]
                    n371 = Concatenate Strings(w1346, "\t", "min: Move ") -> (w1349:string)
                    n372 = call "GetAxisValuesII (SubVI).vi"("read buffer"=w1364) -> ("Array"=w1361:dbl[])  [unwired: 10 in]
                    n373 = call "GetAxisValuesII (SubVI).vi"("read buffer"=w1359) -> ("Array"=w1356:dbl[])  [unwired: 10 in]
                    n374 = for {
                      tunnel: w1361 -> [w1377] mode=indexing
                      tunnel: w1356 -> [w1376] mode=indexing
                      shift-right: [w1378] -> w1347
                      shift-left: w1349 -> [w1379]
                      i -> [w1374]
                      n375 = Subtract(x=w1377, y=w1376) -> (x-y=w1371:dbl)
                      n376 = Divide(x=w1371, y=10.0) -> (x/y=w1373:dbl)
                      n377 = case shown="0, Default" w1374 {
                        tunnel: ["X " "Y " "Z "] -> w1370
                        frame 0, Default {
                        }
                        frame 1 {
                        }
                        frame 2 {
                        }
                      }
                      n378 = Number To Fractional String(number=w1373, precision (6)=i16 2 ("Genauigkeit (6)")) -> (F-format string=w1369:string)  [unwired: 2 in]
                      n379 = Concatenate Strings(w1379, w1370, w1369, "\t") -> (w1378:string)
                    }
                    n380 = Insert Into Array(array=w1366, new element=w1347) -> (w1367:string[])  [unwired: 1 in]
                  }
                }
              }
            }
            n381 = case shown="True" w1165 {
              frame False {
              }
              frame True {
                n382 = Build Array(0.0, 0.0) -> (w1301:dbl[])
                n383 = Build Array(0.0, 30.0) -> (w1302:dbl[])
                n384 = Bundle(w1302, w1301) -> (w1300:cluster{dbl[], dbl[]})  [unwired: 1 in]
                n385 = Build Array(w1300, w1300, w1300, w1300) -> (w1298:cluster{dbl[], dbl[]}[])
                n386 = local write "dV-SISE channel 1"(w1298) -> ()
                n387 = local write "deltaV SISE 1"(w1298) -> ()
                n388 = local write "deltaV SISE 2"(w1298) -> ()
                n389 = local write "V-SISE channel 1"(w1298) -> ()
                n390 = local write "Enable change position 0"(FALSE) -> ()
                n391 = local write "V-SISE channel 2"(w1298) -> ()
                n392 = local write "dV-SISE channel 2"(w1298) -> ()
                n393 = local write "Voltage channel 1"(w1298) -> ()
                n394 = local write "Voltage channel 2"(w1298) -> ()
              }
            }
            n395 = Greater?(x=w1196, y=w1114) -> (0:w1199:bool)
            n396 = case shown="True" w1199 {
              tunnel: w1197 -> [w1383 w1389]
              tunnel: w1114 -> [_ w1391]
              tunnel: w1158 -> [w1385 w1394]
              tunnel: w1196 -> [_ w1393]
              tunnel: [w1384 w1390] -> w1190
              tunnel: w1195 -> [_ w1388]
              frame False {
                n397 = case shown="False" w1385 {
                  tunnel: [w1386 0.0] -> w1384
                  tunnel: w1383 -> [w1386 _]
                  frame False {
                  }
                  frame True {
                  }
                }
              }
              frame True {
                n398 = Divide(x=w1389, y=w1393) -> (x/y=w1392:dbl)
                n399 = case shown="False" w1394 {
                  tunnel: w1391 -> [w1397 w1401]
                  tunnel: w1392 -> [w1396 w1405]
                  tunnel: [w1395 w1399] -> w1390
                  tunnel: w1389 -> [_ w1404]
                  tunnel: w1388 -> [_ w1398]
                  frame False {
                    n400 = Multiply(x=w1396, y=w1397) -> (x*y=w1395:dbl)
                  }
                  frame True {
                    n401 = Multiply(x=w1405, y=w1401) -> (x*y=w1406:dbl)
                    n402 = Equal?(x=w1398, y=0) -> (x = y?=w1403:bool)
                    n403 = Subtract(x=w1404, y=w1406) -> (x-y=w1400:dbl)
                    n404 = case shown="True" w1403 {
                      tunnel: [w1407 0.0] -> w1399
                      tunnel: w1400 -> [w1407 _]
                      frame False {
                      }
                      frame True {
                      }
                    }
                  }
                }
              }
            }
            n405 = case shown="False" w1110 {
              tunnel: w1113 -> [w1241 _]
              tunnel: [w1240 10.0] -> w1112
              frame False {
                n406 = Less?(x=w1241, y=7.0) -> (x < y?=w1239:bool)
                n407 = case shown="False" w1239 {
                  tunnel: w1241 -> [w1243 _]
                  tunnel: [w1243 7.0] -> w1240
                  frame False {
                  }
                  frame True {
                  }
                }
              }
              frame True {
              }
            }
            n408 = Build Array(w1121, w1190) -> (w1146:dbl[])
            n409 = Wait (ms)(milliseconds to wait=w1112) -> ()  [unwired: 1 out]
            n410 = Insert Into Array(array=w1146, new element=w1147) -> (w1148:dbl[])  [unwired: 1 in]
            n411 = Insert Into Array(array=w1146, new element=w1154) -> (w1124:dbl[])  [unwired: 1 in]
            n412 = for {
              tunnel: w1124 -> [w1248] mode=indexing
              shift-right: [w1247] -> w1152
              shift-left: "" -> [w1249]
              n413 = Number To Fractional String(number=w1248) -> (F-format string=w1250:string)  [unwired: 3 in]
              n414 = Concatenate Strings(w1249, w1250, "\t") -> (w1247:string)
            }
            n415 = case shown="False" "Stop measurent" {
              tunnel: [w1614 TRUE] -> w1144
              tunnel: w1224 -> [w1614 _]
              frame False {
              }
              frame True {
              }
            }
            "Stop recording" <- w1144
            n416 = Insert Into Array(array=w1156, new element=w1148) -> (w1161:dbl[][])  [unwired: 2 in]
            n417 = Concatenate Strings(w1152, w1174, "\r\n") -> (w1175:string)
            n418 = Write to Text File(file (use dialog)=w1178, text=w1175, error in=w1179) -> (refnum out=w1177:refnum<file>, error out=w1176:errorcluster)  [unwired: 1 in, 1 out]
          }
          "Stop recording 2" <- w1064
          n419 = Bundle(w1070, w1082) -> (w1081:cluster{string[], dbl[][]})  [unwired: 1 in]
          n420 = Enqueue Element(queue=w1087, element=w1081, error in (no error)=w1086) -> (queue out=w1085:refnum<queue>, error out=w1084:errorcluster)  [unwired: 1 in, 1 out]
        }
        n421 = while {
          tunnel: w547 -> [w626]
          tunnel: w540 -> [w606]
          shift-right: [w578] -> _
          shift-left: w541 -> [w621]
          shift-right: [w595] -> _
          shift-left: dbl[][] [] -> [w596]
          shift-right: [w597] -> _
          shift-left: string[] ["Time, Event mark"] -> [w598]
          tunnel: w513 -> [w568]
          i -> [w577]
          stop <- w622 stop-if-true
          # "Replace time axis"
          # "Calculate average values"
          # "Determine dV"
          # "Combine traces for regression"
          n422 = local read "Stop recording"() -> (w623:bool)
          n423 = Dequeue Element(queue=w626) -> (element=w601:cluster{string[], dbl[][]}, error out=w625:errorcluster)  [unwired: 2 in, 2 out]
          n424 = local read "Start fit (% of rec. period)"() -> (w610:dbl)
          n425 = Greater Or Equal?(x=w577, y=2) -> (x >= y?=w588:bool)
          n426 = Unbundle By Name(w625) -> ("status"=w624:bool)
          n427 = Or(x=w624, y=w623) -> (x .or. y?=w622:bool)
          n428 = Unbundle(w601) -> (w599:string[], w600:dbl[][])
          n429 = Multiply(x=w606, y=w610) -> (x*y=w591:dbl)
          n430 = Multiply(x=w606, y=100.0) -> (x*y=w592:dbl)
          n431 = Multiply(x=w606, y=100.0) -> (x*y=w619:dbl)
          n432 = Multiply(x=w606, y=200.0) -> (x*y=w618:dbl)
          n433 = Array Subset(array=w621, index (row)=w619, length (row)=w618) -> (w615:dbl[][])  [unwired: 2 in]
          n434 = Delete From Array(array=w600, index (col)=1 ("Deaktivierter Index (Spalte)")) -> (array with subset deleted=w614:dbl[][])  [unwired: 2 in, 1 out]
          n435 = Insert Into Array(array=w615, new element=w614) -> (w578:dbl[][])  [unwired: 2 in]
          n436 = local read "Start fit (% of rec. period)"() -> (w607:dbl)
          n437 = Multiply(x=w606, y=w607) -> (x*y=w604:dbl)
          n438 = Multiply(x=w606, y=100.0) -> (x*y=w603:dbl)
          n439 = Add(x=w604, y=w603) -> (x+y=w605:dbl)
          n440 = Subtract(x=w603, y=w604) -> (x-y=w593:dbl)
          n441 = Array Subset(array=w578, index (row)=w605, length (row)=w593) -> (w580:dbl[][])  [unwired: 2 in]
          n442 = Transpose 2D Array(2D array=w580) -> (transposed array=w579:dbl[][])
          n443 = for {
            tunnel: w579 -> [w715] mode=indexing
            shift-right: [w714] -> w583
            shift-left: dbl[] [] -> [w713]
            n444 = Add Array Elements(numeric array=w715) -> (sum=w716:dbl)
            n445 = Array Size(array=w715) -> (size(s)=w717:i32)
            n446 = Divide(x=w716, y=w717) -> (x/y=w712:dbl)
            n447 = Insert Into Array(array=w713, new element=w712) -> (w714:dbl[])  [unwired: 1 in]
          }
          n448 = Index Array(array=w578, index (col)=0 ("Deaktivierter Index (Spalte)")) -> (element=w587:dbl[])  [unwired: 1 in]
          n449 = Index Array(array=w583, index=0 ("Index (Spalte)")) -> (element=w585:dbl)
          n450 = for {
            tunnel: w585 -> [w1056]
            shift-right: [w1059] -> w611
            shift-left: dbl[] [] -> [w1058]
            tunnel: w587 -> [w1055] mode=indexing
            n451 = Subtract(x=w1055, y=w1056) -> (x-y=w1057:dbl)
            n452 = Insert Into Array(array=w1058, new element=w1057) -> (w1059:dbl[])  [unwired: 1 in]
          }
          n453 = Replace Array Subset(array=w578, new element=w611, index (col)=0 ("Deaktivierter Index (Spalte)")) -> (w584:dbl[][])  [unwired: 1 in]
          n454 = for {
            N: 2 -> [_]
            tunnel: w584 -> [w642]
            tunnel: w592 -> [w641]
            tunnel: w591 -> [w640]
            tunnel: w588 -> [w636]
            tunnel: w577 -> [w634]
            shift-right: [w633] -> w581
            shift-left: dbl[] [] -> [w632]
            i -> [w639]
            n455 = flat-sequence {
              tunnel: w642 -> [w653]
              tunnel: w640 -> [w654]
              tunnel: w641 -> [w661]
              tunnel: [w658] -> w644
              tunnel: [w655] -> w643
              tunnel: w635 -> [w649]
              tunnel: w644 -> [w685]
              tunnel: w643 -> [w691]
              tunnel: w634 -> [w686]
              tunnel: [w674] -> w631
              tunnel: [w673] -> w637
              frame #0 {
                n456 = Subtract(x=w661, y=w654) -> (x-y=w667:dbl)
                n457 = Multiply(x=w661, y=2.0) -> (x*y=w664:dbl)
                n458 = Add(x=w654, y=w664) -> (x+y=w672:dbl)
                n459 = Add(x=w654, y=w661) -> (x+y=w671:dbl)
                n460 = Array Subset(array=w653, index (row)=w654, length (row)=w667) -> (w669:dbl[][])  [unwired: 2 in]
                n461 = Array Subset(array=w653, index (row)=w672, length (row)=w667) -> (w670:dbl[][])  [unwired: 2 in]
                n462 = Array Subset(array=w653, index (row)=w671, length (row)=w667) -> (w662:dbl[][])  [unwired: 2 in]
                n463 = Insert Into Array(array=w669, new element=w670) -> (w665:dbl[][])  [unwired: 2 in]
                n464 = Index Array(array=w662, index (col)=w649) -> (element=w652:dbl[])  [unwired: 1 in]
                n465 = Index Array(array=w665, index (col)=0 ("disabled index (col)")) -> (element=w660:dbl[])  [unwired: 1 in]
                n466 = Index Array(array=w662, index (col)=0 ("disabled index (col)")) -> (element=w651:dbl[])  [unwired: 1 in]
                n467 = Index Array(array=w665, index (col)=w649) -> (element=w659:dbl[])  [unwired: 1 in]
                n468 = call <vilib>:"Linear Fit.vi"("Y"=w659, "X"=w660) -> ("Best Linear Fit"=w650:dbl[], "slope"=w657:dbl, "intercept"=w656:dbl)  [unwired: 9 in, 2 out]
                n469 = Build Array(w657, w656) -> (w655:dbl[])
                n470 = Bundle(w660, w659, "Best Linear Fit"=w650, w651, w652) -> (w658:T8)  [unwired: 1 in]
              }
              frame #1 {
                n471 = Unbundle(w685) -> (w696:dbl[], w697:dbl[])  [unwired: 3 out]
                n472 = Divide(x=w686, y=2 ("x")) -> (x/y=w687:dbl)
                n473 = Index Array(array=w691, index=0 ("Index")) -> (element=w698:dbl)
                n474 = Index Array(array=w691, index=1 ("Index")) -> (element=w690:dbl)
                n475 = Unbundle(w685) -> (w682:dbl[], w684:dbl[], "Best Linear Fit"=w681:dbl[], w680:dbl[], w678:dbl[])
                n476 = Round To Nearest(number=w687) -> (nearest integer value=w688:dbl)
                n477 = Absolute Value(x=w698) -> (abs(x)=w703:dbl)
                n478 = Equal?(x=w688, y=w687) -> (x = y?=w693:bool)
                n479 = Divide(x=w703, y=1000.0) -> (x/y=w705:dbl)
                n480 = Bundle(w682, w684) -> (w683:cluster{dbl[], dbl[]})  [unwired: 1 in]
                n481 = Bundle(w682, "Best Linear Fit"=w681) -> (w677:cluster{dbl[], "Best Linear Fit":dbl[]})  [unwired: 1 in]
                n482 = Bundle(w680, w678) -> (w675:cluster{dbl[], dbl[]})  [unwired: 1 in]
                n483 = Subtract(x=w698, y=w705) -> (x-y=w702:dbl)
                n484 = Add(x=w698, y=w705) -> (x+y=w701:dbl)
                n485 = Bundle(w702, w701, -inf, inf) -> (w700:cluster{dbl, dbl, dbl, dbl})  [unwired: 1 in]
                n486 = call <vilib>:"Linear Fit.vi"("Y"=w697, "X"=w696, "parameter bounds"=w700) -> ("Best Linear Fit"=w679:dbl[], "intercept"=w689:dbl)  [unwired: 8 in, 3 out]
                n487 = Subtract(x=w690, y=w689) -> (x-y=w694:dbl)
                n488 = Bundle(w680, "Best Linear Fit"=w679) -> (w676:cluster{dbl[], "Best Linear Fit":dbl[]})  [unwired: 1 in]
                n489 = case shown="True" w693 {
                  tunnel: w694 -> [w708 w710]
                  tunnel: [w708 w711] -> w674
                  frame False {
                  }
                  frame True {
                    n490 = Multiply(x=-1.0, y=w710) -> (x*y=w711:dbl)
                  }
                }
                n491 = Build Array(w683, w677, w676, w675) -> (w673:cluster{dbl[], "Best Linear Fit":dbl[]}[])
              }
            }
            n492 = Add(x=1, y=w639) -> (x+y=w635:i32)
            n493 = case shown="True" w636 {
              tunnel: w637 -> [_ w646]
              tunnel: w635 -> [_ w645]
              frame False {
              }
              frame True {
                n494 = case shown="0, Default" w645 {
                  tunnel: w646 -> [_ w647 w648]
                  frame 0, Default {
                  }
                  frame 1 {
                    "deltaV SISE 1" <- w647
                  }
                  frame 2 {
                    "deltaV SISE 2" <- w648
                  }
                }
              }
            }
            n495 = Insert Into Array(array=w632, new element=w631) -> (w633:dbl[])  [unwired: 1 in]
          }
          n496 = Insert Into Array(array=w583, index=3 ("Index"), new element=w581) -> (w570:dbl[])
          n497 = Index Array(array=w570, index=0 ("Index")) -> (element=w572:dbl)
          n498 = Divide(x=w572, y=60.0) -> (x/y=w571:dbl)
          n499 = Replace Array Subset(array=w570, new element=w571, index=0 ("Index")) -> (w569:dbl[])
          n500 = case shown="True" w588 {
            tunnel: w596 -> [w627 w630]
            tunnel: [w627 w629] -> w595
            tunnel: w569 -> [_ w628]
            frame False {
            }
            frame True {
              n501 = Insert Into Array(array=w630, new element=w628) -> (w629:dbl[][])  [unwired: 2 in]
            }
          }
          n502 = while {
            tunnel: w595 -> [w724]
            tunnel: w599 -> [w741]
            tunnel: w598 -> [w740]
            tunnel: [w731] -> w597
            tunnel: w577 -> [w730]
            tunnel: w577 -> [w725]
            tunnel: w568 -> [w723]
            i -> [w775]
            stop <- w720 stop-if-true
            n503 = for {
              tunnel: w741 -> [w1035] mode=indexing
              shift-right: [w1032] -> w726
              shift-left: TRUE -> [w1036]
              n504 = Equal?(x=w1035, y="") -> (x = y?=w1033:bool)
              n505 = case shown="True" w1033 {
                tunnel: w1036 -> [_ w1038]
                tunnel: [FALSE w1038] -> w1032
                frame False {
                }
                frame True {
                }
              }
            }
            n506 = Wait (ms)(milliseconds to wait=u32 100 ("Zu wartende ms")) -> ()  [unwired: 1 out]
            n507 = Multiply(x="Zoom from end", y=-1.0) -> (x*y=w759:dbl)
            n508 = Add(x="Zoom from start", y=w759) -> (x+y=w770:dbl)
            n509 = feedback #4() -> (w765:dbl)  [unwired: 1 in]
            n510 = Greater Or Equal?(x=w770, y=0.0) -> (x >= y?=w768:bool)
            n511 = Less?(x=w730, y=2) -> (x < y?=w728:bool)
            n512 = case shown="True" w768 {
              tunnel: "Zoom from start" -> [w1047 w1050]
              tunnel: [w1046 w1050] -> w766
              tunnel: w765 -> [w1046 w1052]
              tunnel: "Zoom from end" -> [_ w1049]
              tunnel: [w1047 w1050] -> w758
              tunnel: [w1045 w1048] -> w757
              tunnel: "Zoom from end" -> [w1045 w1048]
              frame False {
              }
              frame True {
                n513 = Not Equal?(x=w1052, y=w1050) -> (x != y?=w1051:bool)
                n514 = case shown="False" w1051 {
                  tunnel: w1050 -> [_ w1054]
                  tunnel: w1049 -> [w1053 _]
                  frame False {
                    n515 = local write "Zoom from start"(w1053) -> ()
                  }
                  frame True {
                    n516 = local write "Zoom from end"(w1054) -> ()
                  }
                }
              }
            }
            n517 = feedback-in #4(w766) -> ()
            n518 = Or(x=w726, y=w728) -> (x .or. y?=w727:bool)
            n519 = case shown="False" w727 {
              tunnel: w740 -> [w1028 w1031]
              tunnel: [w1030 w1031] -> w731
              tunnel: w741 -> [w1029 _]
              frame False {
                n520 = Insert Into Array(array=w1028, new element=w1029) -> (w1030:string[])  [unwired: 1 in]
              }
              frame True {
              }
            }
            n521 = Array Size(array=w731) -> (size(s)=w737:i32)
            n522 = Array Subset(array=w731, index=1 ("Index")) -> (w745:string[])  [unwired: 1 in]
            n523 = Subtract(x=w757, y=w758) -> (x-y=w764:dbl)
            n524 = Divide(x=w737, y=10) -> (x/y=w735:dbl)
            n525 = for {
              tunnel: w745 -> [w1041] mode=indexing
              shift-right: [w1044] -> w743
              shift-left: dbl[] [] -> [w1043]
              n526 = Match Pattern(string=w1041, regular expression="\t") -> (before substring=w1039:string)  [unwired: 1 in, 3 out]
              n527 = Fract/Exp String To Number(string=w1039) -> (number=w1042:dbl)  [unwired: 3 in, 1 out]
              n528 = Insert Into Array(array=w1043, new element=w1042) -> (w1044:dbl[])  [unwired: 1 in]
            }
            n529 = Index Array(array=w724, index (col)=0 ("Deaktivierter Index (Spalte)")) -> (element=w772:dbl[])  [unwired: 1 in]
            n530 = Multiply(x=w735, y="Bildlaufleiste") -> (x*y=w733:dbl)
            n531 = Divide(x=w758, y=100.0) -> (x/y=w760:dbl)
            n532 = Divide(x=w764, y=100.0) -> (x/y=w761:dbl)
            n533 = Array Size(array=w772) -> (size(s)=w754:i32)
            n534 = Array Subset(array=w731, index=w733) -> (w732:string[])  [unwired: 1 in]
            n535 = Multiply(x=w754, y=w760) -> (x*y=w750:dbl)
            n536 = Multiply(x=w754, y=w761) -> (x*y=w753:dbl)
            n537 = Index Array(array=w723, index="TC 3") -> (element=w722:bool)
            n538 = Add(x=w753, y=2.0) -> (x+y=w751:dbl)
            n539 = Subtract(x=w750, y=2.0) -> (x-y=w748:dbl)
            n540 = for {
              shift-right: [w1026] -> w738
              shift-left: "" -> [w1027]
              tunnel: w732 -> [w1024] mode=indexing
              n541 = Concatenate Strings(w1027, w1024, "\r") -> (w1026:string)
            }
            "?" <- w738
            n542 = Array Subset(array=w724, index (row)=w748, length (row)=w751) -> (w744:dbl[][])  [unwired: 2 in]
            n543 = case shown="\"V channel #1\"" "TC 3" {
              tunnel: w744 -> [w787 w867 w979 w990]
              tunnel: w743 -> [w785 w866 w947 w993]
              tunnel: w725 -> [w784 w863 w944 w985]
              tunnel: w722 -> [w781 w862 w943 w984]
              frame "SISE channel #1", Default {
                n544 = Greater Or Equal?(x=w784, y=2) -> (x >= y?=w782:bool)
                n545 = And(x=w782, y=w781) -> (x .and. y?=w780:bool)
                n546 = Index Array(array=w787, index (col)=0 ("disabled index (col)")) -> (element=w790:dbl[])  [unwired: 1 in]
                n547 = Index Array(array=w787, index (col)=1 ("disabled index (col)")) -> (element=w789:dbl[])  [unwired: 1 in]
                n548 = Index Array(array=w787, index (col)=3 ("disabled index (col)")) -> (element=w786:dbl[])  [unwired: 1 in]
                n549 = stacked-sequence {
                  tunnel: w790 -> [w794 w833]
                  tunnel: w789 -> [w813 _]
                  tunnel: w785 -> [w795 w832]
                  tunnel: w786 -> [_ w831]
                  tunnel: w780 -> [w793 w827]
                  frame #0 {
                    n550 = Array Max & Min(array=w794) -> (max value=w805:dbl, min value=w804:dbl)  [unwired: 2 out]
                    n551 = Divide(x="Range limit\nS1.1 (mV)", y=2.0) -> (x/y=w823:dbl)
                    n552 = Divide(x="Range limit\nS1.1 (mV)", y=2.05) -> (x/y=w824:dbl)
                    n553 = Add(x="Base line\nS1.1 (mV)", y=w823) -> (x+y=w796:dbl)
                    n554 = Subtract(x="Base line\nS1.1 (mV)", y=w823) -> (x-y=w797:dbl)
                    n555 = Subtract(x="Base line\nS1.1 (mV)", y=w824) -> (x-y=w803:dbl)
                    n556 = call "EventstoGraph (SubVI).vi"("Numerisch 2"=w804, "Array 3"=w795, "Numerisch"=w805, "Array (Eingang)"=dbl[][] [], "Numerisch 3"=w803) -> ("Array (Ausgang)"=w807:dbl[][])  [unwired: 6 in]
                    n557 = Array Max & Min(array=w794) -> (max value=w819:dbl, min value=w820:dbl)  [unwired: 2 out]
                    n558 = call "GraphLimit01.vi"("Numeric 2"=w797, "Numeric"=w796, "Array in"=w813, "Array 3"=dbl[] []) -> ("Array out"=w812:dbl[])  [unwired: 7 in]
                    n559 = Build Array("Base line\nS1.1 (mV)", "Base line\nS1.1 (mV)") -> (w816:dbl[])
                    n560 = Build Array(w819, w820) -> (w817:dbl[])
                    n561 = Build Array(w796, w797) -> (w818:dbl[])
                    n562 = Index Array(array=w807, index (col)=0 ("Index (Zeile)")) -> (element=w808:dbl[])  [unwired: 1 in]
                    n563 = Index Array(array=w807, index (col)=1 ("Index (Zeile)")) -> (element=w806:dbl[])  [unwired: 1 in]
                    n564 = Bundle(w817, w818) -> (w800:cluster{dbl[], dbl[]})  [unwired: 1 in]
                    n565 = Bundle(w817, w816) -> (w801:cluster{dbl[], dbl[]})  [unwired: 1 in]
                    n566 = Bundle(w794, "Array out"=w812) -> (w799:cluster{dbl[], "Array out":dbl[]})  [unwired: 1 in]
                    n567 = Bundle("Array (Ausgang)"=w808, "Array (Ausgang)"=w806) -> (w798:T9)  [unwired: 1 in]
                    n568 = Build Array(w801, w800, w799, w798) -> (w802:T10)
                    n569 = case shown="True" w793 {
                      tunnel: w802 -> [_ w826]
                      frame False {
                      }
                      frame True {
                        "V-SISE channel 1" <- w826
                      }
                    }
                  }
                  frame #1 {
                    n570 = Array Max & Min(array=w833) -> (max value=w842:dbl, min value=w841:dbl)  [unwired: 2 out]
                    n571 = Divide(x="Range limit\nS1.2 mV", y=2.0) -> (x/y=w858:dbl)
                    n572 = Divide(x="Range limit\nS1.2 mV", y=2.05) -> (x/y=w859:dbl)
                    n573 = Add(x="Base line \nS1.2 (mV)", y=w858) -> (x+y=w834:dbl)
                    n574 = Subtract(x="Base line \nS1.2 (mV)", y=w858) -> (x-y=w835:dbl)
                    n575 = Subtract(x="Base line \nS1.2 (mV)", y=w859) -> (x-y=w840:dbl)
                    n576 = call "EventstoGraph (SubVI).vi"("Numerisch 2"=w841, "Array 3"=w832, "Numerisch"=w842, "Array (Eingang)"=dbl[][] [], "Numerisch 3"=w840) -> ("Array (Ausgang)"=w844:dbl[][])  [unwired: 6 in]
                    n577 = Array Max & Min(array=w833) -> (max value=w854:dbl, min value=w855:dbl)  [unwired: 2 out]
                    n578 = call "GraphLimit01.vi"("Numeric 2"=w835, "Numeric"=w834, "Array in"=w831, "Array 3"=dbl[] []) -> ("Array out"=w849:dbl[])  [unwired: 7 in]
                    n579 = Build Array("Base line \nS1.2 (mV)", "Base line \nS1.2 (mV)") -> (w851:dbl[])
                    n580 = Build Array(w854, w855) -> (w852:dbl[])
                    n581 = Build Array(w834, w835) -> (w853:dbl[])
                    n582 = Index Array(array=w844, index (col)=0 ("Index (Zeile)")) -> (element=w845:dbl[])  [unwired: 1 in]
                    n583 = Index Array(array=w844, index (col)=1 ("Index (Zeile)")) -> (element=w843:dbl[])  [unwired: 1 in]
                    n584 = Bundle(w852, w853) -> (w838:cluster{dbl[], dbl[]})  [unwired: 1 in]
                    n585 = Bundle(w852, w851) -> (w839:cluster{dbl[], dbl[]})  [unwired: 1 in]
                    n586 = Bundle(w833, "Array out"=w849) -> (w837:cluster{dbl[], "Array out":dbl[]})  [unwired: 1 in]
                    n587 = Bundle("Array (Ausgang)"=w845, "Array (Ausgang)"=w843) -> (w836:T9)  [unwired: 1 in]
                    n588 = Build Array(w839, w838, w837, w836) -> (w828:T10)
                    n589 = case shown="True" w827 {
                      tunnel: w828 -> [_ w860]
                      frame False {
                      }
                      frame True {
                        "dV-SISE channel 1" <- w860
                      }
                    }
                  }
                }
              }
              frame "SISE channel #2" {
                n590 = Greater Or Equal?(x=w863, y=2) -> (x >= y?=w865:bool)
                n591 = And(x=w865, y=w862) -> (x .and. y?=w861:bool)
                n592 = Index Array(array=w867, index (col)=0 ("disabled index (col)")) -> (element=w871:dbl[])  [unwired: 1 in]
                n593 = Index Array(array=w867, index (col)=2 ("disabled index (col)")) -> (element=w872:dbl[])  [unwired: 1 in]
                n594 = Index Array(array=w867, index (col)=4 ("disabled index (col)")) -> (element=w873:dbl[])  [unwired: 1 in]
                n595 = stacked-sequence {
                  tunnel: w871 -> [w875 w914]
                  tunnel: w872 -> [w894 _]
                  tunnel: w866 -> [w876 w913]
                  tunnel: w873 -> [_ w912]
                  tunnel: w861 -> [w874 w908]
                  frame #0 {
                    n596 = Array Max & Min(array=w875) -> (max value=w886:dbl, min value=w885:dbl)  [unwired: 2 out]
                    n597 = Divide(x="Range limit\nS2.1 (mV)", y=2.0) -> (x/y=w904:dbl)
                    n598 = Divide(x="Range limit\nS2.1 (mV)", y=2.05) -> (x/y=w905:dbl)
                    n599 = Add(x="Base line\nS2.1 (mV)", y=w904) -> (x+y=w877:dbl)
                    n600 = Subtract(x="Base line\nS2.1 (mV)", y=w904) -> (x-y=w878:dbl)
                    n601 = Subtract(x="Base line\nS2.1 (mV)", y=w905) -> (x-y=w884:dbl)
                    n602 = call "EventstoGraph (SubVI).vi"("Numerisch 2"=w885, "Array 3"=w876, "Numerisch"=w886, "Array (Eingang)"=dbl[][] [], "Numerisch 3"=w884) -> ("Array (Ausgang)"=w888:dbl[][])  [unwired: 6 in]
                    n603 = Array Max & Min(array=w875) -> (max value=w900:dbl, min value=w901:dbl)  [unwired: 2 out]
                    n604 = call "GraphLimit01.vi"("Numeric 2"=w878, "Numeric"=w877, "Array in"=w894, "Array 3"=dbl[] []) -> ("Array out"=w893:dbl[])  [unwired: 7 in]
                    n605 = Build Array("Base line\nS2.1 (mV)", "Base line\nS2.1 (mV)") -> (w897:dbl[])
                    n606 = Build Array(w900, w901) -> (w898:dbl[])
                    n607 = Build Array(w877, w878) -> (w899:dbl[])
                    n608 = Index Array(array=w888, index (col)=0 ("Index (Zeile)")) -> (element=w889:dbl[])  [unwired: 1 in]
                    n609 = Index Array(array=w888, index (col)=1 ("Index (Zeile)")) -> (element=w887:dbl[])  [unwired: 1 in]
                    n610 = Bundle(w898, w899) -> (w881:cluster{dbl[], dbl[]})  [unwired: 1 in]
                    n611 = Bundle(w898, w897) -> (w882:cluster{dbl[], dbl[]})  [unwired: 1 in]
                    n612 = Bundle(w875, "Array out"=w893) -> (w880:cluster{dbl[], "Array out":dbl[]})  [unwired: 1 in]
                    n613 = Bundle("Array (Ausgang)"=w889, "Array (Ausgang)"=w887) -> (w879:T9)  [unwired: 1 in]
                    n614 = Build Array(w882, w881, w880, w879) -> (w883:T10)
                    n615 = case shown="True" w874 {
                      tunnel: w883 -> [_ w907]
                      frame False {
                      }
                      frame True {
                        "V-SISE channel 2" <- w907
                      }
                    }
                  }
                  frame #1 {
                    n616 = Array Max & Min(array=w914) -> (max value=w923:dbl, min value=w922:dbl)  [unwired: 2 out]
                    n617 = Divide(x="Range limit\nS2.2 (mV)", y=2.0) -> (x/y=w939:dbl)
                    n618 = Divide(x="Range limit\nS2.2 (mV)", y=2.05) -> (x/y=w940:dbl)
                    n619 = Add(x="Base line \nS2.2 (mV)", y=w939) -> (x+y=w915:dbl)
                    n620 = Subtract(x="Base line \nS2.2 (mV)", y=w939) -> (x-y=w916:dbl)
                    n621 = Subtract(x="Base line \nS2.2 (mV)", y=w940) -> (x-y=w921:dbl)
                    n622 = call "EventstoGraph (SubVI).vi"("Numerisch 2"=w922, "Array 3"=w913, "Numerisch"=w923, "Array (Eingang)"=dbl[][] [], "Numerisch 3"=w921) -> ("Array (Ausgang)"=w925:dbl[][])  [unwired: 6 in]
                    n623 = Array Max & Min(array=w914) -> (max value=w935:dbl, min value=w936:dbl)  [unwired: 2 out]
                    n624 = call "GraphLimit01.vi"("Numeric 2"=w916, "Numeric"=w915, "Array in"=w912, "Array 3"=dbl[] []) -> ("Array out"=w930:dbl[])  [unwired: 7 in]
                    n625 = Build Array("Base line \nS2.2 (mV)", "Base line \nS2.2 (mV)") -> (w932:dbl[])
                    n626 = Build Array(w935, w936) -> (w933:dbl[])
                    n627 = Build Array(w915, w916) -> (w934:dbl[])
                    n628 = Index Array(array=w925, index (col)=0 ("Index (Zeile)")) -> (element=w926:dbl[])  [unwired: 1 in]
                    n629 = Index Array(array=w925, index (col)=1 ("Index (Zeile)")) -> (element=w924:dbl[])  [unwired: 1 in]
                    n630 = Bundle(w933, w934) -> (w919:cluster{dbl[], dbl[]})  [unwired: 1 in]
                    n631 = Bundle(w933, w932) -> (w920:cluster{dbl[], dbl[]})  [unwired: 1 in]
                    n632 = Bundle(w914, "Array out"=w930) -> (w918:cluster{dbl[], "Array out":dbl[]})  [unwired: 1 in]
                    n633 = Bundle("Array (Ausgang)"=w926, "Array (Ausgang)"=w924) -> (w917:T9)  [unwired: 1 in]
                    n634 = Build Array(w920, w919, w918, w917) -> (w909:T10)
                    n635 = case shown="True" w908 {
                      tunnel: w909 -> [_ w941]
                      frame False {
                      }
                      frame True {
                        "dV-SISE channel 2" <- w941
                      }
                    }
                  }
                }
              }
              frame "V channel #1" {
                n636 = Greater Or Equal?(x=w944, y=2) -> (x >= y?=w946:bool)
                n637 = And(x=w946, y=w943) -> (x .and. y?=w942:bool)
                n638 = Index Array(array=w979, index (col)=0 ("disabled index (col)")) -> (element=w948:dbl[])  [unwired: 1 in]
                n639 = Index Array(array=w979, index (col)=5 ("disabled index (col)")) -> (element=w949:dbl[])  [unwired: 1 in]
                n640 = Array Max & Min(array=w948) -> (max value=w959:dbl, min value=w958:dbl)  [unwired: 2 out]
                n641 = Divide(x="Range limit\nV1 (V)", y=2.0) -> (x/y=w976:dbl)
                n642 = Divide(x="Range limit\nV1 (V)", y=2.05) -> (x/y=w977:dbl)
                n643 = Add(x="Base line\nV1 (V)", y=w976) -> (x+y=w950:dbl)
                n644 = Subtract(x="Base line\nV1 (V)", y=w976) -> (x-y=w951:dbl)
                n645 = Subtract(x="Base line\nV1 (V)", y=w977) -> (x-y=w957:dbl)
                n646 = call "EventstoGraph (SubVI).vi"("Numerisch 2"=w958, "Array 3"=w947, "Numerisch"=w959, "Array (Eingang)"=dbl[][] [], "Numerisch 3"=w957) -> ("Array (Ausgang)"=w961:dbl[][])  [unwired: 6 in]
                n647 = Array Max & Min(array=w948) -> (max value=w972:dbl, min value=w973:dbl)  [unwired: 2 out]
                n648 = call "GraphLimit01.vi"("Numeric 2"=w951, "Numeric"=w950, "Array in"=w949, "Array 3"=dbl[] []) -> ("Array out"=w966:dbl[])  [unwired: 7 in]
                n649 = Build Array("Base line\nV1 (V)", "Base line\nV1 (V)") -> (w969:dbl[])
                n650 = Build Array(w972, w973) -> (w970:dbl[])
                n651 = Build Array(w950, w951) -> (w971:dbl[])
                n652 = Index Array(array=w961, index (col)=0 ("Index (Zeile)")) -> (element=w962:dbl[])  [unwired: 1 in]
                n653 = Index Array(array=w961, index (col)=1 ("Index (Zeile)")) -> (element=w960:dbl[])  [unwired: 1 in]
                n654 = Bundle(w970, w971) -> (w954:cluster{dbl[], dbl[]})  [unwired: 1 in]
                n655 = Bundle(w970, w969) -> (w955:cluster{dbl[], dbl[]})  [unwired: 1 in]
                n656 = Bundle(w948, "Array out"=w966) -> (w953:cluster{dbl[], "Array out":dbl[]})  [unwired: 1 in]
                n657 = Bundle("Array (Ausgang)"=w962, "Array (Ausgang)"=w960) -> (w952:T9)  [unwired: 1 in]
                n658 = Build Array(w955, w954, w953, w952) -> (w956:T10)
                n659 = case shown="True" w942 {
                  tunnel: w956 -> [_ w982]
                  frame False {
                  }
                  frame True {
                    "Voltage channel 1" <- w982
                  }
                }
              }
              frame "V channel #2" {
                n660 = Greater Or Equal?(x=w985, y=2) -> (x >= y?=w986:bool)
                n661 = And(x=w986, y=w984) -> (x .and. y?=w983:bool)
                n662 = Index Array(array=w990, index (col)=0 ("disabled index (col)")) -> (element=w988:dbl[])  [unwired: 1 in]
                n663 = Index Array(array=w990, index (col)=6 ("disabled index (col)")) -> (element=w989:dbl[])  [unwired: 1 in]
                n664 = Array Max & Min(array=w988) -> (max value=w1003:dbl, min value=w1002:dbl)  [unwired: 2 out]
                n665 = Divide(x="Range limit\nV2 (V)", y=2.0) -> (x/y=w1020:dbl)
                n666 = Divide(x="Range limit\nV2 (V)", y=2.05) -> (x/y=w1021:dbl)
                n667 = Add(x="Base line\nV2 (V)", y=w1020) -> (x+y=w994:dbl)
                n668 = Subtract(x="Base line\nV2 (V)", y=w1020) -> (x-y=w995:dbl)
                n669 = Subtract(x="Base line\nV2 (V)", y=w1021) -> (x-y=w1001:dbl)
                n670 = call "EventstoGraph (SubVI).vi"("Numerisch 2"=w1002, "Array 3"=w993, "Numerisch"=w1003, "Array (Eingang)"=dbl[][] [], "Numerisch 3"=w1001) -> ("Array (Ausgang)"=w1005:dbl[][])  [unwired: 6 in]
                n671 = Array Max & Min(array=w988) -> (max value=w1016:dbl, min value=w1017:dbl)  [unwired: 2 out]
                n672 = call "GraphLimit01.vi"("Numeric 2"=w995, "Numeric"=w994, "Array in"=w989, "Array 3"=dbl[] []) -> ("Array out"=w1010:dbl[])  [unwired: 7 in]
                n673 = Build Array("Base line\nV2 (V)", "Base line\nV2 (V)") -> (w1013:dbl[])
                n674 = Build Array(w1016, w1017) -> (w1014:dbl[])
                n675 = Build Array(w994, w995) -> (w1015:dbl[])
                n676 = Index Array(array=w1005, index (col)=0 ("Index (Zeile)")) -> (element=w1006:dbl[])  [unwired: 1 in]
                n677 = Index Array(array=w1005, index (col)=1 ("Index (Zeile)")) -> (element=w1004:dbl[])  [unwired: 1 in]
                n678 = Bundle(w1014, w1015) -> (w998:cluster{dbl[], dbl[]})  [unwired: 1 in]
                n679 = Bundle(w1014, w1013) -> (w999:cluster{dbl[], dbl[]})  [unwired: 1 in]
                n680 = Bundle(w988, "Array out"=w1010) -> (w997:cluster{dbl[], "Array out":dbl[]})  [unwired: 1 in]
                n681 = Bundle("Array (Ausgang)"=w1006, "Array (Ausgang)"=w1004) -> (w996:T9)  [unwired: 1 in]
                n682 = Build Array(w999, w998, w997, w996) -> (w1000:T10)
                n683 = case shown="True" w983 {
                  tunnel: w1000 -> [_ w1023]
                  frame False {
                  }
                  frame True {
                    "Voltage channel 2" <- w1023
                  }
                }
              }
            }
            n684 = local read "Record period (round at 5s)"() -> (w774:dbl)
            n685 = local read "Stop recording 2"() -> (w718:bool)
            n686 = Multiply(x=w774, y=10.0) -> (x*y=w778:dbl)
            n687 = Subtract(x=w778, y=10.0) -> (x-y=w776:dbl)
            n688 = Greater Or Equal?(x=w775, y=w776) -> (x >= y?=w719:bool)
            n689 = Or(x=w718, y=w719) -> (x .or. y?=w720:bool)
          }
        }
        n690 = Unbundle(w517) -> ("status"=w554:bool, "code"=w553:i32, "source"=w552:string)
        n691 = call <vilib>:"DAQmx Stop Task.vi"("task/channels in"=w518, "error in"=w517) -> ()  [unwired: 12 in, 2 out]
        n692 = Close File(refnum=w515, error in=w516) -> ()  [unwired: 2 out]
        n693 = Unbundle(w516) -> ("status"=w533:bool, "code"=w532:i32, "source"=w531:string)
        n694 = Bundle("task out"=w518, "status"=w554, "code"=w553, "source"=w552) -> (w551:T5)  [unwired: 1 in]
        n695 = Bundle("refnum out"=w515, "status"=w533, "code"=w532, "source"=w531) -> (w530:T4)  [unwired: 1 in]
        n696 = Release Queue(queue=w549, error in (no error)=w548) -> ()  [unwired: 1 in, 3 out]
      }
      frame 2 {
        n697 = while {
          tunnel: w1618 -> [w1626]
          tunnel: [w1625] -> w1617
          stop <- w1629 stop-if-true
          n698 = Wait (ms)(milliseconds to wait=u32 100 ("Zu wartende ms")) -> ()  [unwired: 1 out]
          n699 = case shown="True" "Stop programm" {
            tunnel: w1626 -> [w1631 _]
            tunnel: [w1631 TRUE] -> w1625
            frame False {
            }
            frame True {
            }
          }
          n700 = Or(x="New measurement", y="Stop programm") -> (x .or. y?=w1629:bool)
        }
      }
    }
    "Registerkarte" <- w27
  }
